vi "Hardware Configuration Dialog.vi"(6 "Update UI Values?":bool, 8 "error in (no error)":errorcluster, 9 "Function":enum16{"Initialize", "Action"}(ring)=enum."Action", 10 "Hardware Status":T1={"Parameter Analyzer"={"Configuration"={"Parameter Analyzer VISA Session"="COM1", "Sweeping Time Parameters"={"Integration Time"=0, "Short Integration Time (s)"=1.0, "Long Integration Time (s)"=0.0, "Wait Time Parameter"=1.0}, "Acquisition Mode"=enum."Sweeping Mode", "Status Polling Time (ms)"=1000, "Comment"="Test VI", "SMU 1 - Sweeping"={"Start / Offset"=0.0, "Stop / Ratio"=1.0, "Step \n(linear only)"=0.01, "Compliance"=0.1, "Power \nCompliance"=0.0, "Mode"=0, "Function"=0, "Sweep Mode"=FALSE}, "SMU 2 - Sweeping"={"Start / Offset"=0.0, "Stop / Ratio"=1.0, "Step \n(linear only)"=0.01, "Compliance"=0.1, "Power \nCompliance"=0.0, "Mode"=0, "Function"=0, "Sweep Mode"=FALSE}, "SMU 3 - Sweeping"={"Start / Offset"=0.0, "Stop / Ratio"=1.0, "Step \n(linear only)"=0.01, "Compliance"=0.1, "Power \nCompliance"=0.0, "Mode"=0, "Function"=0, "Sweep Mode"=FALSE}, "SMU 4 - Sweeping"={"Start / Offset"=0.0, "Stop / Ratio"=1.0, "Step \n(linear only)"=0.01, "Compliance"=0.1, "Power \nCompliance"=0.0, "Mode"=0, "Function"=0, "Sweep Mode"=FALSE}, "Sweep Spacing"=0, "Range"=0, "SMU1 - Sampling"={"Source"=10.0, "Compliance"=1e-05, "Mode"=0, "Function"=FALSE}, "SMU2 - Sampling"={"Source"=10.0, "Compliance"=1e-05, "Mode"=0, "Function"=FALSE}, "SMU3 - Sampling"={"Source"=10.0, "Compliance"=1e-05, "Mode"=0, "Function"=FALSE}, "SMU4 - Sampling"={"Source"=0.1, "Compliance"=60.0, "Mode"=10, "Function"=FALSE}, "Sampling Time Parameters"={"Initial Interval (s)"=0.1, "Number of Samples"=60, "Total Sampling Time (s)"=10.0, "Hold Time (s)"=0.0, "Sampling Mode"=0, "Sampling Time"=0}, "Stop Condition"={"Enable Delay (s)"=0.0, "Name"="", "Threshold"=0.0, "num. of events"=1, "Event"=0, "Stop Condition Enable"=FALSE}}, "Refnums"={"Status"=refnum, "Electrical Measurement"=refnum, "Plots"={"Plot List"=refnum, "Voltage Plot"=refnum, "Current Plot"=refnum, "IV Characteristic"=refnum, "dI/dV-V Characteristic"=refnum}, "HP Integration Time"=refnum, "VISA"=refnum, "Sweeping Time Parameters"=refnum, "Acquisition Mode"=refnum, "SMU 1 - Sweeping"=refnum, "SMU 2 - Sweeping"=refnum, "SMU 3 - Sweeping"=refnum, "SMU 4 - Sweeping"=refnum, "Sweep Spacing"=refnum, "Range"=refnum, "SMU1 - Sampling"=refnum, "SMU2 - Sampling"=refnum, "SMU3 - Sampling"=refnum, "SMU4 - Sampling"=refnum, "Sampling Time Parameters"=refnum, "Stop Condition"=refnum, "Instrument Status"=refnum}, "Initialization"={"Update Visa Session"=FALSE, "Configure Integration Time"=FALSE, "Configure Acquisition Mode"=FALSE, "Update Refnums"=FALSE}}, "Swithing Matrix"={"Configuration"={"Switching Matrix VISA Session"="GPIB0::18::INSTR", "Connections"=[{"Connections"=[FALSE, FALSE, FALSE, FALSE, FALSE, FALSE, FALSE, FALSE, FALSE, FALSE, FALSE, FALSE], "Connection Type"=enum."Disconnected"}, {"Connections"=[FALSE, FALSE, FALSE, FALSE, FALSE, FALSE, FALSE, FALSE, FALSE, FALSE, FALSE, FALSE], "Connection Type"=enum."Disconnected"}, {"Connections"=[FALSE, FALSE, FALSE, FALSE, FALSE, FALSE, FALSE, FALSE, FALSE, FALSE, FALSE, FALSE], "Connection Type"=enum."Disconnected"}, {"Connections"=[FALSE, FALSE, FALSE, FALSE, FALSE, FALSE, FALSE, FALSE, FALSE, FALSE, FALSE, FALSE], "Connection Type"=enum."Disconnected"}, {"Connections"=[FALSE, FALSE, FALSE, FALSE, FALSE, FALSE, FALSE, FALSE, FALSE, FALSE, FALSE, FALSE], "Connection Type"=enum."Disconnected"}, {"Connections"=[FALSE, FALSE, FALSE, FALSE, FALSE, FALSE, FALSE, FALSE, FALSE, FALSE, FALSE, FALSE], "Connection Type"=enum."Disconnected"}, {"Connections"=[FALSE, FALSE, FALSE, FALSE, FALSE, FALSE, FALSE, FALSE, FALSE, FALSE, FALSE, FALSE], "Connection Type"=enum."Disconnected"}, {"Connections"=[FALSE, FALSE, FALSE, FALSE, FALSE, FALSE, FALSE, FALSE, FALSE, FALSE, FALSE, FALSE], "Connection Type"=enum."Disconnected"}]}, "Refnums"={"Connections"=refnum, "Instrument Status"=refnum}, "Initialization"={"Update Visa Session"=FALSE, "Update Refnums"=FALSE}}, "Stress Control"={"Configuration"={"Stress Control VISA Session"="StrainMotor", "Axis"=0, "Motion"=0, "Destination (°)"=0.0, "Speed (°/s)"=4.0, "Position (°)"=25.0}, "Refnums"={"Instrument Status"=refnum, "Position"=refnum, "Mecahnism Motion"=refnum, "Destination"=refnum, "Apply Stress"=refnum, "Stop"=refnum, "Stress Control VISA"=refnum}, "Initialization"={"Update Visa Session"=FALSE, "Update Configuration"=FALSE, "Update Refnums"=FALSE, "Get Position"=FALSE}}, "Optical Spectrometer"={"Configuration"={"Laser Settings"={"Laser Wavelength"=enum."784 nm", "Neutral Density Filter"=enum."50%"}, "Spectrometer Settings"={"Confocal Hole Size (µm)"=150.0, "Grating"=2, "Detector"=enum."InGaAs Array"}, "Acquisition Settings"={"Acquisition Mode"=enum."Multi-Window", "Spectal Position (nm)"=632.0, "From (nm)"=735.0, "To (nm)"=3.0, "Integration Time (s)"=3.0, "Number of Accumulations"=3, "AutoScanning"=FALSE, "Spike Removal"=FALSE}, "Path"=path "C:/07 - Prizes and Awards/Marie Curie Prize/Reply Editors Final NCOMMS(10).docx"}, "Refnums"={"Instrument Status"=refnum, "Optical Spectrum Plot"={"Plot List"=refnum, "Optical Spectrum vs Energy"=refnum, "Optical Spectrum vs Wavelength"=refnum, "Optical Spectrum vs Raman Shift"=refnum, "Detector Temperature"=refnum}, "Laser"=refnum, "Filter"=refnum, "Laser ON?"=refnum, "Hole"=refnum, "Grating"=refnum, "Detector"=refnum, "Acquisition Mode"=refnum, "Spectal Position"=refnum, "From"=refnum, "To"=refnum, "Integration Time"=refnum, "Accumulations"=refnum, "AutoScanning"=refnum, "Spike Removal"=refnum, "Acquisition Mode Panel"=refnum}, "Initialization"={"Connect"=FALSE, "Update Refnums"=FALSE, "Get Configuration"=FALSE}}, "Switches & Mirrors"={"Configuration"={"Relay VISA Session"="COM1", "Switches"={"Laser"=FALSE, "Video"=FALSE}, "Delays (ms)"={"Laser"=500, "Video"=1500}}, "Refnums"={"Instrument Status"=refnum, "Laser"=refnum, "Video"=refnum, "Relay VISA"=refnum}, "Initialize"={"Update Refnums"=FALSE, "Connect"=FALSE, "Set Configuration"=FALSE}}, "Camera"={"Configuration"={"Settings"={"Pixel clock"=20, "Frame rate"=30.0, "Exposure time"=33.21525, "Master Gain"=0, "Red Gain"=0, "Green Gain"=0, "Blue Gain"=0, "Auto Gain"=FALSE, "White-balance"=FALSE, "Color Correction"=FALSE}}, "Refnums"={"Pixel Clock"=refnum, "Frame Rate"=refnum, "Exposure Time"=refnum, "Master Gain"=refnum, "Red Gain"=refnum, "Green Gain"=refnum, "Blue Gain"=refnum, "Auto Gain"=refnum, "Auto White-balance"=refnum, "Color Correction"=refnum, "Image"=refnum, "Video Button"=refnum, "Instrument Status"=refnum}, "Initialization"={"Connect"=FALSE, "Update Refnums"=FALSE, "Acquiring?"=FALSE}}, "XYZ Stage"={"Configuration"={"Connection Settings"={"Tango VISA"="", "Baudrate"=57600, "Show Protocol?"=FALSE}, "Manual Control"={"North"=FALSE, "South"=FALSE, "West"=FALSE, "East"=FALSE, "Up"=FALSE, "Down"=FALSE, "Stop"=FALSE, "XY Step"=0.0, "Z step"=0.0}, "Coordinate Control"={"Motion Mode"=enum."Absolute", "Destination [mm]"=[]}}, "Refnums"={"Instrument Status"=refnum, "Position"=refnum, "Manual Control"=refnum, "Up"=refnum, "Down"=refnum, "North"=refnum, "South"=refnum, "East"=refnum, "West"=refnum, "Stop"=refnum, "Limits"=refnum}, "Initialization"={"Update Visa Session"=FALSE, "Set To Default"=FALSE, "Get Status"=FALSE, "Update Refnums"=FALSE}}, "AutoFocus"={"Configuration"={"Matching Criteria"={"Minimum Score"=700.0, "Color Score Weight"=700.0, "Minimum Contrast"=50, "Match Mode"=0, "Match Feature Mode"=0, "Subpixel Accuracy"=TRUE, "Color Sensitivity"=1, "Search Strategy"=1}, "Z Scan Parameters"={"Z Range"=1380.0, "Resolution"=5000.0, "Initial Direction"=enum."Up", "Focus Threshold"=0.1, "Ascent Constant"=0.1}, "Displacement"=50.0, "Transformation Matrix"=[]}, "Refnums"={"Instrument Status"=refnum, "Matching Criteria"=refnum, "Z Scan Parameters"=refnum, "Distance"=refnum, "Transformation Matrix"=refnum, "Match and Edge"={"Image"=refnum, "Target"=refnum, "Edge"=refnum, "Target Data"=refnum}, "Matching Curves"=refnum, "Tracking"=refnum, "Focus"=refnum, "Find Focus"=refnum, "Set Target"=refnum, "Link Stage & Camera"=refnum, "Align"=refnum}, "Initialize"={"Update Refnums"=FALSE, "Allocate Image Memory"=FALSE, "Set Match Criteria"=FALSE, "Link Stage & Camera"=FALSE, "Set Target"=FALSE, "Find Target"=FALSE}}} {"AutoFocus"."Configuration"."Displacement" scale=1.0..1000.0; "AutoFocus"."Configuration"."Z Scan Parameters"."Focus Threshold" min=0.0 max=1000.0 step=1.0 format="%#_2f"; "AutoFocus"."Configuration"."Z Scan Parameters"."Ascent Constant" min=0.0 max=1000.0 step=1.0 format="%#_2f"; "AutoFocus"."Configuration"."Z Scan Parameters"."Resolution" min=0.0 max=1.0 step=0.01 format="%_2g"; "AutoFocus"."Configuration"."Z Scan Parameters"."Z Range" format="%_3g"; "AutoFocus"."Configuration"."Matching Criteria"."Match Mode" items=["Shift Invariant", "Rotation Invariant"]; "AutoFocus"."Configuration"."Matching Criteria"."Match Feature Mode" items=["Color and Shape", "Color", "Shape"]; "AutoFocus"."Configuration"."Matching Criteria"."Color Sensitivity" items=["Low Sensitivity", "Medium Sensitivity", "High Sensitivity"]; "AutoFocus"."Configuration"."Matching Criteria"."Search Strategy" items=["Conservative", "Balance", "Aggressive", "Very Aggressive"]; "XYZ Stage"."Configuration"."Manual Control"."Z step" scale=0.1..10.0; "XYZ Stage"."Configuration"."Manual Control"."XY Step" scale=0.1..1000.0; "Camera"."Configuration"."Settings"."Blue Gain" min=0 max=100 scale=0.0..100.0; "Camera"."Configuration"."Settings"."Green Gain" min=0 max=100 scale=0.0..100.0; "Camera"."Configuration"."Settings"."Red Gain" min=0 max=100 scale=0.0..100.0; "Camera"."Configuration"."Settings"."Master Gain" min=0 max=100 scale=0.0..100.0; "Camera"."Configuration"."Settings"."Exposure time" min=0.101625 max=159.246375 step=0.101625 scale=0.101625..159.246375 scale format="%#.3g"; "Camera"."Configuration"."Settings"."Frame rate" min=2.7455631699174137 max=6.2675785993528725 step=0.000101625 scale=2.7455631699174137..6.2675785993528725 scale format="%^#_3g"; "Camera"."Configuration"."Settings"."Pixel clock" min=5 max=43 scale=5.0..43.0; "Optical Spectrometer"."Configuration"."Spectrometer Settings"."Grating" items=["1800 l/mm", "150 l/mm"]; "Stress Control"."Configuration"."Axis" min=1 max=3; "Stress Control"."Configuration"."Position (°)" format="%.6g"; "Stress Control"."Configuration"."Speed (°/s)" min=0.0 max=4.0 format="%.6f"; "Stress Control"."Configuration"."Destination (°)" min=-2000000000.0 max=2000000000.0 format="%.6f"; "Stress Control"."Configuration"."Motion" items=["Absolute", "Relative"]; "Parameter Analyzer"."Configuration"."Stop Condition"."Event" items=["Value > Threshold", "Value < Threshold", "| Value | > | Threshold |", "| Value | < | Threshold |"]; "Parameter Analyzer"."Configuration"."Stop Condition"."Threshold" format="%^.2e"; "Parameter Analyzer"."Configuration"."Stop Condition"."Enable Delay (s)" format="%.1f"; "Parameter Analyzer"."Configuration"."Sampling Time Parameters"."Sampling Time" items=["Auto (linear only)", "No Limit", "Set Limit"]; "Parameter Analyzer"."Configuration"."Sampling Time Parameters"."Sampling Mode" items=["Linear", "Log10", "Log25", "Log50", "Thinned Out"]; "Parameter Analyzer"."Configuration"."Sampling Time Parameters"."Hold Time (s)" format="%.4f"; "Parameter Analyzer"."Configuration"."Sampling Time Parameters"."Total Sampling Time (s)" format="%.1f"; "Parameter Analyzer"."Configuration"."Sampling Time Parameters"."Initial Interval (s)" format="%^.3e"; "Parameter Analyzer"."Configuration"."SMU 4 - Sweeping"."Function" items=["Disabled", "Var 1", "Var 2", "Var 1'", "Constant"]; "Parameter Analyzer"."Configuration"."SMU 4 - Sweeping"."Mode" items=["V", "I", "V pulse", "I  pulse", "Common"]; "Parameter Analyzer"."Configuration"."SMU 4 - Sweeping"."Power \nCompliance" format="%^.2e"; "Parameter Analyzer"."Configuration"."SMU 4 - Sweeping"."Compliance" format="%^.2e"; "Parameter Analyzer"."Configuration"."SMU 4 - Sweeping"."Step \n(linear only)" format="%^.4e"; "Parameter Analyzer"."Configuration"."SMU 4 - Sweeping"."Stop / Ratio" format="%^.4e"; "Parameter Analyzer"."Configuration"."SMU 4 - Sweeping"."Start / Offset" format="%^.4e"; "Parameter Analyzer"."Configuration"."SMU 3 - Sweeping"."Function" items=["Disabled", "Var 1", "Var 2", "Var 1'", "Constant"]; "Parameter Analyzer"."Configuration"."SMU 3 - Sweeping"."Mode" items=["V", "I", "V pulse", "I  pulse", "Common"]; "Parameter Analyzer"."Configuration"."SMU 3 - Sweeping"."Power \nCompliance" format="%^.2e"; "Parameter Analyzer"."Configuration"."SMU 3 - Sweeping"."Compliance" format="%^.2e"; "Parameter Analyzer"."Configuration"."SMU 3 - Sweeping"."Step \n(linear only)" format="%^.4e"; "Parameter Analyzer"."Configuration"."SMU 3 - Sweeping"."Stop / Ratio" format="%^.4e"; "Parameter Analyzer"."Configuration"."SMU 3 - Sweeping"."Start / Offset" format="%^.4e"; "Parameter Analyzer"."Configuration"."SMU 2 - Sweeping"."Function" items=["Disabled", "Var 1", "Var 2", "Var 1'", "Constant"]; "Parameter Analyzer"."Configuration"."SMU 2 - Sweeping"."Mode" items=["V", "I", "V pulse", "I  pulse", "Common"]; "Parameter Analyzer"."Configuration"."SMU 2 - Sweeping"."Power \nCompliance" format="%^.2e"; "Parameter Analyzer"."Configuration"."SMU 2 - Sweeping"."Compliance" format="%^.2e"; "Parameter Analyzer"."Configuration"."SMU 2 - Sweeping"."Step \n(linear only)" format="%^.4e"; "Parameter Analyzer"."Configuration"."SMU 2 - Sweeping"."Stop / Ratio" format="%^.4e"; "Parameter Analyzer"."Configuration"."SMU 2 - Sweeping"."Start / Offset" format="%^.4e"; "Parameter Analyzer"."Configuration"."SMU 1 - Sweeping"."Function" items=["Disabled", "Var 1", "Var 2", "Var 1'", "Constant"]; "Parameter Analyzer"."Configuration"."SMU 1 - Sweeping"."Mode" items=["V", "I", "V pulse", "I  pulse", "Common"]; "Parameter Analyzer"."Configuration"."SMU 1 - Sweeping"."Power \nCompliance" format="%^.2e"; "Parameter Analyzer"."Configuration"."SMU 1 - Sweeping"."Compliance" format="%^.2e"; "Parameter Analyzer"."Configuration"."SMU 1 - Sweeping"."Step \n(linear only)" format="%^.4e"; "Parameter Analyzer"."Configuration"."SMU 1 - Sweeping"."Stop / Ratio" format="%^.4e"; "Parameter Analyzer"."Configuration"."SMU 1 - Sweeping"."Start / Offset" format="%^.4e"; "Parameter Analyzer"."Configuration"."Sweeping Time Parameters"."Long Integration Time (s)" scale=0.02..2.0; "Parameter Analyzer"."Configuration"."Sweeping Time Parameters"."Short Integration Time (s)" scale=8e-05..0.00192; "Parameter Analyzer"."Configuration"."Sweeping Time Parameters"."Integration Time" items=["Short", "Long"]; "Parameter Analyzer"."Configuration"."Sweeping Time Parameters"."Wait Time Parameter" format="%.1f"; "Parameter Analyzer"."Configuration"."SMU4 - Sampling"."Mode" items=["V", "I", "Common"]; "Parameter Analyzer"."Configuration"."SMU4 - Sampling"."Compliance" format="%^.2e"; "Parameter Analyzer"."Configuration"."SMU4 - Sampling"."Source" format="%^.3e"; "Parameter Analyzer"."Configuration"."SMU3 - Sampling"."Mode" items=["V", "I", "Common"]; "Parameter Analyzer"."Configuration"."SMU3 - Sampling"."Compliance" format="%^.2e"; "Parameter Analyzer"."Configuration"."SMU3 - Sampling"."Source" format="%^.3e"; "Parameter Analyzer"."Configuration"."SMU2 - Sampling"."Mode" items=["V", "I", "Common"]; "Parameter Analyzer"."Configuration"."SMU2 - Sampling"."Compliance" format="%^.2e"; "Parameter Analyzer"."Configuration"."SMU2 - Sampling"."Source" format="%^.3e"; "Parameter Analyzer"."Configuration"."SMU1 - Sampling"."Mode" items=["V", "I", "Common"]; "Parameter Analyzer"."Configuration"."SMU1 - Sampling"."Compliance" format="%^.2e"; "Parameter Analyzer"."Configuration"."SMU1 - Sampling"."Source" format="%^.3e"; "Parameter Analyzer"."Configuration"."Range" items=["auto", "fixed", "limited"]; "Parameter Analyzer"."Configuration"."Sweep Spacing" items=["linear", "log 10", "log 25", "log 50"]}, 11 "Instrument Steps In":T58) -> (0 "error out":errorcluster, 2 "Instrument Steps Out":T58)   [LabVIEW 2014]
uses:
  Instrument Steps.ctl
  Action.ctl
  Instrument List.ctl
  support/Status of All Instruments.ctl
  Hardware Control/Parameter Analyzer/Parameter Analyzer Data.ctl
  Hardware Control/Parameter Analyzer/Parameter Analyzer Config.ctl
  Hardware Control/Parameter Analyzer/Parameter Analyzer Integration Parameters.ctl
  Hardware Control/Parameter Analyzer/Parameter Analyzer SMU Sweeping.ctl
  Hardware Control/Parameter Analyzer/Parameter Analyzer Sweep Spacing.ctl
  Hardware Control/Parameter Analyzer/Parameter Analyzer SMU Range.ctl
  Hardware Control/Parameter Analyzer/Parameter Analyzer SMU Sampling.ctl
  Hardware Control/Parameter Analyzer/Parameter Analyzer Sampling Parameters.ctl
  Hardware Control/Parameter Analyzer/Parameter Analyzer Stop Sampling Conditions.ctl
  Hardware Control/Parameter Analyzer/Parameter Analyzer Refnums.ctl
  Plot Data/Electrical Data Plot Refnums.ctl
  Hardware Control/Parameter Analyzer/Parameter Analyzer Initialization.ctl
  Hardware Control/Switching Matrix/Switching Matrix Data.ctl
  Hardware Control/Switching Matrix/Switching Matrix Config.ctl
  Hardware Control/Switching Matrix/Switching Matrix Refnums.ctl
  Hardware Control/Switching Matrix/Switching Matrix Initialization.ctl
  Hardware Control/Stress Control/StressControl Data.ctl
  Hardware Control/Stress Control/StressControl Config.ctl
  Hardware Control/Stress Control/StressControl Refnums.ctl
  Hardware Control/Stress Control/StressControl Initialization.ctl
  Hardware Control/Spectrometer/Spectrometer Data.ctl
  Hardware Control/Spectrometer/Spectrometer Config.ctl
  Hardware Control/Spectrometer/Laser Settings.ctl
  Hardware Control/Spectrometer/Laser.ctl
  Hardware Control/Spectrometer/Filter.ctl
  Hardware Control/Spectrometer/Grating Detector Settings.ctl
  Hardware Control/Spectrometer/Grating.ctl
  Hardware Control/Spectrometer/Detector.ctl
  Hardware Control/Spectrometer/Acquisition Settings.ctl
  Hardware Control/Spectrometer/Spectrometer Refnum.ctl
  Plot Data/Optical Spectrum Plot Refnum.ctl
  Hardware Control/Spectrometer/Spectrometer Initialization.ctl
  Hardware Control/Switches and Mirrors/SwitchesMirrors Data.ctl
  Hardware Control/Switches and Mirrors/SwitchesMirrors Config.ctl
  Hardware Control/Switches and Mirrors/SwitchesMirrors Status.ctl
  Hardware Control/Switches and Mirrors/SwitchesMirrors Refnum.ctl
  support/Instrument Status.ctl
  Hardware Control/Switches and Mirrors/SwitchesMirrors Initialize.ctl
  Hardware Control/Camera/Camera Data.ctl
  Hardware Control/Camera/Camera Config.ctl
  Hardware Control/Camera/Camera Settings.ctl
  Hardware Control/Camera/Camera Refnums.ctl
  Hardware Control/Camera/Camera Initialization.ctl
  Hardware Control/XYZ Stage/XYZ Data.ctl
  Hardware Control/XYZ Stage/XYZ Config.ctl
  Hardware Control/XYZ Stage/XYZ Connection Settings.ctl
  Hardware Control/XYZ Stage/XYZ Stage Control.ctl
  Hardware Control/XYZ Stage/XYZ Coordinate Control.ctl
  Hardware Control/XYZ Stage/XYZ Refnums.ctl
  <instrlib>/Tango Drivers/Labview/SubVIs/Axis_Switch.ctl
  Hardware Control/XYZ Stage/XYZ Initialization.ctl
  Hardware Control/Autofocus/AutoFocus Data.ctl
  Hardware Control/Autofocus/AutoFocus Config.ctl
  Hardware Control/Autofocus/ZScan.ctl
  <vilib>/Analysis/Matrix/Datatypes/RealMatrix.ctl
  Hardware Control/Autofocus/AutoFocus Refnums.ctl
  Hardware Control/Autofocus/Target Refnums.ctl
  Hardware Control/Autofocus/AutoFocus Initialize.ctl
  <vilib>/Analysis/Matrix/NI_Matrix.lvlib
panel:
  in  "Unused Functions":enum32{"Delete Step"}(tab)
  in  "Step Index":i32 min=0 max=6 step=1
  in  "Delete Instrument Step":bool
  in  "Action":T61(tab)
  in  "Measure Optoelectronic":bool
  in  "Focus":bool
  in  "Wavelength":T25=enum."365 nm"
  in  "Power":T62(ring)
  in  "Detector":T29=enum."Silicon CCD"
  in  "Grating":T28 items=["1800 l/mm", "150 l/mm"]
  in  "Confocal Hole Size (µm)":dbl=70.0
  in  "Acquisition Mode":enum32{"Single Window", "Multi Window"}(tab)
  in  "Spectal Position (nm)":dbl=363.99945438000003
  in  "From (nm)":dbl=632.0
  in  "To (nm)":dbl=1000.0
  in  "Spectrum Integration Time (s)":dbl=3.0 caption="Integration Time (s)"
  in  "Number of Accumulations":i32=3
  in  "AutoScanning":bool
  in  "Spike Removal":bool
  in  "Configure Spectrometer":bool
  in  "Measure Optical Spectrum":bool
  in  "Switching Matrix Connections":T63(array[cluster])=[{"Connections"=[FALSE, FALSE, FALSE, FALSE, FALSE, FALSE, FALSE, FALSE, FALSE, FALSE, FALSE, FALSE], "Connection Type"=enum."Disconnected"}, {"Connections"=[FALSE, FALSE, FALSE, FALSE, FALSE, FALSE, FALSE, FALSE, FALSE, FALSE, FALSE, FALSE], "Connection Type"=enum."Disconnected"}, {"Connections"=[FALSE, FALSE, FALSE, FALSE, FALSE, FALSE, FALSE, FALSE, FALSE, FALSE, FALSE, FALSE], "Connection Type"=enum."Disconnected"}, {"Connections"=[FALSE, FALSE, FALSE, FALSE, FALSE, FALSE, FALSE, FALSE, FALSE, FALSE, FALSE, FALSE], "Connection Type"=enum."Disconnected"}, {"Connections"=[FALSE, FALSE, FALSE, FALSE, FALSE, FALSE, FALSE, FALSE, FALSE, FALSE, FALSE, FALSE], "Connection Type"=enum."Disconnected"}, {"Connections"=[FALSE, FALSE, FALSE, FALSE, FALSE, FALSE, FALSE, FALSE, FALSE, FALSE, FALSE, FALSE], "Connection Type"=enum."Disconnected"}, {"Connections"=[FALSE, FALSE, FALSE, FALSE, FALSE, FALSE, FALSE, FALSE, FALSE, FALSE, FALSE, FALSE], "Connection Type"=enum."Disconnected"}, {"Connections"=[FALSE, FALSE, FALSE, FALSE, FALSE, FALSE, FALSE, FALSE, FALSE, FALSE, FALSE, FALSE], "Connection Type"=enum."Disconnected"}]
  in  "Configure Switching Matrix":bool
  in  "Measurement Mode":enum32{"Sweeping Mode", "Sampling Mode"}(tab)
  in  "SMU 4 - Sweeping 2":T64={"Start / Offset"=0.0, "Stop / Ratio"=1.0, "Step \n(linear only)"=0.01, "Compliance"=0.1, "Power \nCompliance"=0.0, "Mode"=4, "Function"=4, "Sweep Mode"=FALSE} caption="SMU 4" {"Function" items=["Disabled", "Var 1", "Var 2", "Var 1'", "Constant"]; "Mode" items=["V", "I", "V pulse", "I  pulse", "Common"]; "Power \nCompliance" format="%^.2e"; "Compliance" format="%^.2e"; "Step \n(linear only)" format="%^.4e"; "Stop / Ratio" format="%^.4e"; "Start / Offset" format="%^.4e"}
  in  "SMU 3 - Sweeping 2":T64={"Start / Offset"=0.0, "Stop / Ratio"=1.0, "Step \n(linear only)"=0.01, "Compliance"=0.1, "Power \nCompliance"=0.0, "Mode"=1, "Function"=4, "Sweep Mode"=FALSE} caption="SMU 3" {"Function" items=["Disabled", "Var 1", "Var 2", "Var 1'", "Constant"]; "Mode" items=["V", "I", "V pulse", "I  pulse", "Common"]; "Power \nCompliance" format="%^.2e"; "Compliance" format="%^.2e"; "Step \n(linear only)" format="%^.4e"; "Stop / Ratio" format="%^.4e"; "Start / Offset" format="%^.4e"}
  in  "SMU 2 - Sweeping 2":T64={"Start / Offset"=0.0, "Stop / Ratio"=1.0, "Step \n(linear only)"=0.01, "Compliance"=0.1, "Power \nCompliance"=0.0, "Mode"=1, "Function"=4, "Sweep Mode"=FALSE} caption="SMU 2" {"Function" items=["Disabled", "Var 1", "Var 2", "Var 1'", "Constant"]; "Mode" items=["V", "I", "V pulse", "I  pulse", "Common"]; "Power \nCompliance" format="%^.2e"; "Compliance" format="%^.2e"; "Step \n(linear only)" format="%^.4e"; "Stop / Ratio" format="%^.4e"; "Start / Offset" format="%^.4e"}
  in  "SMU 1 - Sweeping 2":T64={"Start / Offset"=0.0, "Stop / Ratio"=0.15, "Step \n(linear only)"=0.01, "Compliance"=0.1, "Power \nCompliance"=0.0, "Mode"=0, "Function"=1, "Sweep Mode"=TRUE} caption="SMU 1" {"Function" items=["Disabled", "Var 1", "Var 2", "Var 1'", "Constant"]; "Mode" items=["V", "I", "V pulse", "I  pulse", "Common"]; "Power \nCompliance" format="%^.2e"; "Compliance" format="%^.2e"; "Step \n(linear only)" format="%^.4e"; "Stop / Ratio" format="%^.4e"; "Start / Offset" format="%^.4e"}
  in  "User Integration Time":T65={"Integration Time"=0, "Short Integration Time (s)"=0.0, "Long Integration Time (s)"=0.0, "Wait Time Parameter"=1.0} caption="Input Integration Time" {"Long Integration Time (s)" scale=0.02..2.0; "Short Integration Time (s)" scale=8e-05..0.00192; "Integration Time" items=["Short", "Long"]; "Wait Time Parameter" format="%.1f"}
  in  "Range":u16(ring) items=["auto", "fixed", "limited"]
  in  "Sweep Spacing":u16(ring) items=["linear", "log 10", "log 25", "log 50"]
  in  "SMU4 - Sampling":T66={"Source"=10.0, "Compliance"=1e-05, "Mode"=0, "Function"=FALSE} caption="SMU 4" {"Mode" items=["V", "I", "Common"]; "Compliance" format="%^.2e"; "Source" format="%^.3e"}
  in  "SMU2 - Sampling":T66={"Source"=10.0, "Compliance"=1e-05, "Mode"=0, "Function"=FALSE} caption="SMU 2" {"Mode" items=["V", "I", "Common"]; "Compliance" format="%^.2e"; "Source" format="%^.3e"}
  in  "SMU3 - Sampling":T66={"Source"=10.0, "Compliance"=1e-05, "Mode"=0, "Function"=FALSE} caption="SMU 3" {"Mode" items=["V", "I", "Common"]; "Compliance" format="%^.2e"; "Source" format="%^.3e"}
  in  "SMU1 - Sampling":T66={"Source"=10.0, "Compliance"=1e-05, "Mode"=0, "Function"=FALSE} caption="SMU 1" {"Mode" items=["V", "I", "Common"]; "Compliance" format="%^.2e"; "Source" format="%^.3e"}
  in  "Stop Condition":T67={"Enable Delay (s)"=0.0, "Name"="", "Threshold"=0.0, "num. of events"=1, "Event"=0, "Stop Condition Enable"=FALSE} {"Event" items=["Value > Threshold", "Value < Threshold", "| Value | > | Threshold |", "| Value | < | Threshold |"]; "Threshold" format="%^.2e"; "Enable Delay (s)" format="%.1f"}
  in  "Sampling Parameters":T68={"Initial Interval (s)"=0.1, "Number of Samples"=60, "Total Sampling Time (s)"=10.0, "Hold Time (s)"=0.0, "Sampling Mode"=0, "Sampling Time"=0} {"Sampling Time" items=["Auto (linear only)", "No Limit", "Set Limit"]; "Sampling Mode" items=["Linear", "Log10", "Log25", "Log50", "Thinned Out"]; "Hold Time (s)" format="%.4f"; "Total Sampling Time (s)" format="%.1f"; "Initial Interval (s)" format="%^.3e"}
  in  "Configure Generic Parameter Analyzer":bool
  in  "Measure Parameter Analyzer 1":bool
  in  "Integration Time (s)":dbl(slide)=0.02 min=0.02 max=2.0 scale=8e-05..2.0
  in  "Measurement Type":enum32{"Four Probe", "Two Probe"}(ring)
  in  "Force Mode":enum32{"Voltage", "Current"}(ring)
  in  "Power Compliance":dbl format="%^.2e"
  in  "Compliance":dbl=0.001 format="%^.2e"
  in  "Step Size":dbl=0.001 format="%^.4e"
  in  "Maximum Force":dbl=0.15 format="%^.4e"
  in  "Measure Parameter Analyzer 2":bool
  in  "Configure Two/Four Probe":bool
  in  "Sweep Mode":bool
  # "LICENSED MATERIALS – PROPERTY OF IBM\nCopyright IBM Corp. 2016,\nALL RIGHTS RESERVED"
  # "XY"
  # "Z"
  # "XY"
  # "Z"
  # "Laser Settings"
  # "Spectrometer Settings"
  # "Acquisition Settings"
  # "SMU1"
  # "SMU2"
  # "SMU3"
  # "SMU4"
  # "CH1"
  # "CH2"
  # "CH3"
  # "CH4"
  # "L1"
  # "R1"
  # "L2"
  # "R2"
  # "L3"
  # "R3"
  # "L6"
  # "R6"
  # "L7"
  # "R7"
  # "L8"
  # "R8"
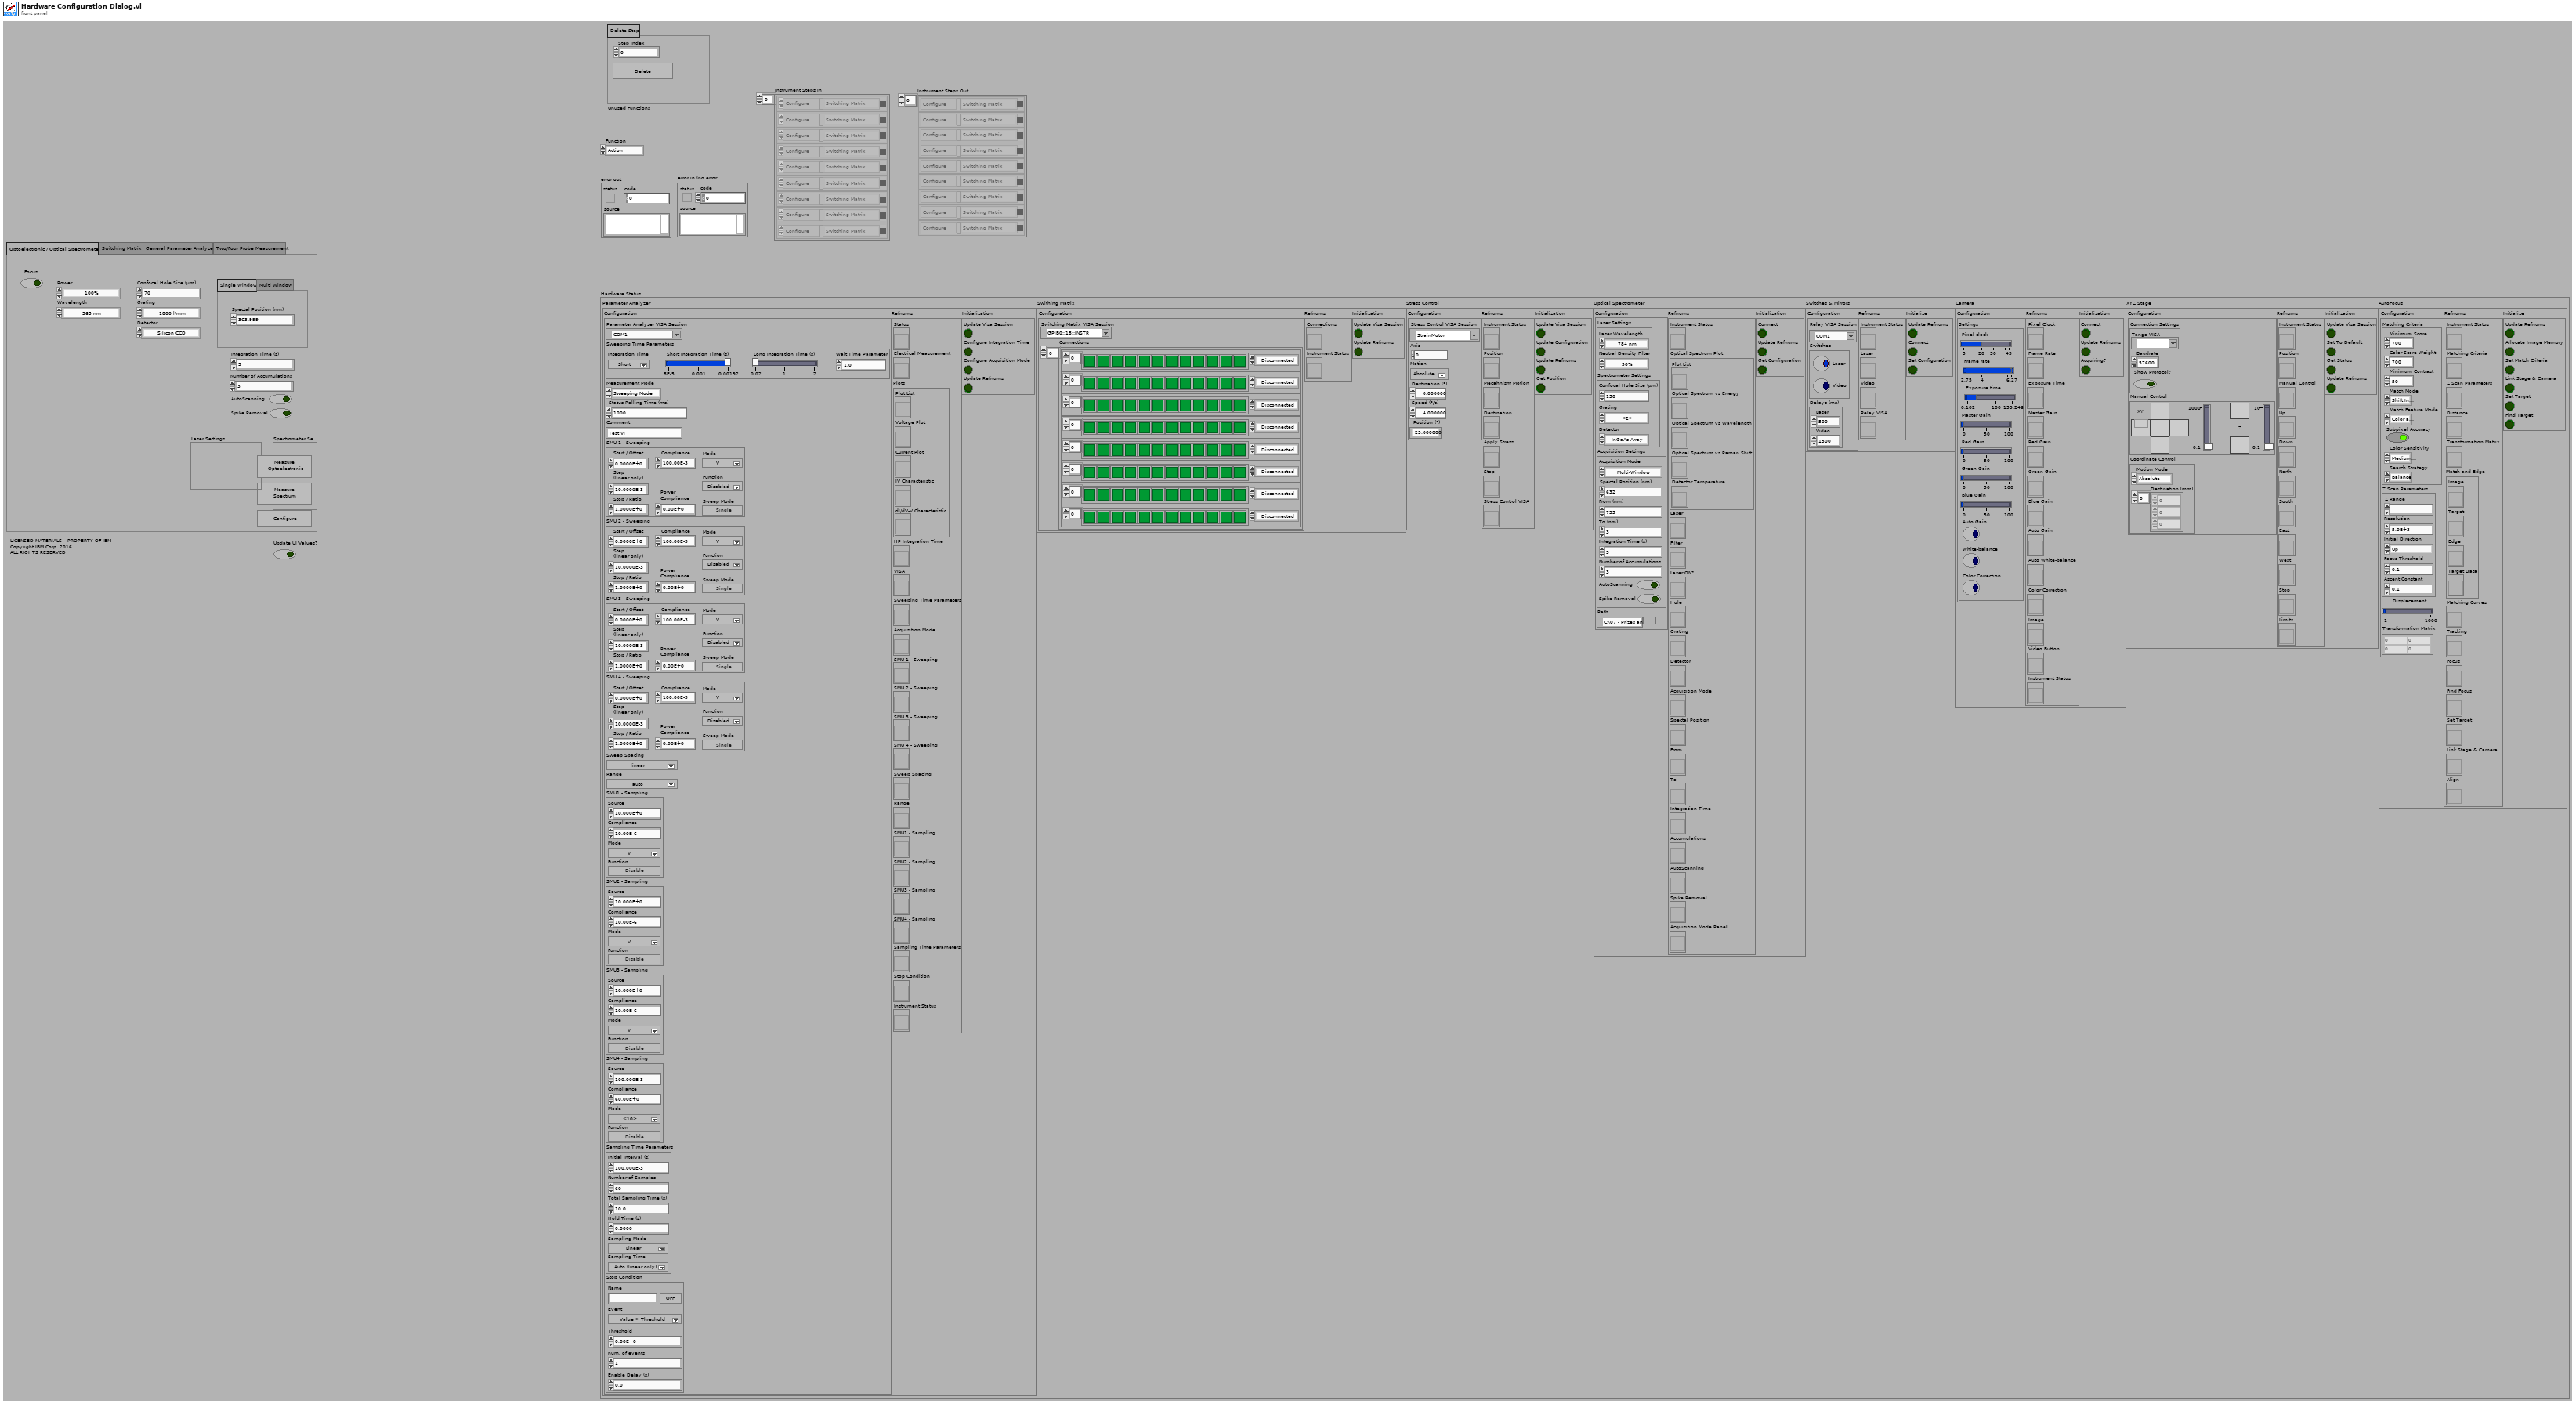
[diagram p1: front panel]
types:
  T1 = typedef "Status of All Instruments.ctl" = cluster{"Parameter Analyzer":T2, "Swithing Matrix":T14, "Stress Control":T18, "Optical Spectrometer":T22, "Switches & Mirrors":T34, "Camera":T39, "XYZ Stage":T44, "AutoFocus":T51}
  T2 = typedef "Parameter Analyzer Data.ctl" = cluster{"Configuration":T3, "Refnums":T11, "Initialization":T13}
  T3 = typedef "Parameter Analyzer Config.ctl" = cluster{"Parameter Analyzer VISA Session":refnum<visa-resource-name>, "Sweeping Time Parameters":T4, "Acquisition Mode":enum32{"Sweeping Mode", "Sampling Mode"}, "Status Polling Time (ms)":u32, "Comment":string, "SMU 1 - Sweeping":T5, "SMU 2 - Sweeping":T5, "SMU 3 - Sweeping":T5, "SMU 4 - Sweeping":T5, "Sweep Spacing":T6, "Range":T7, "SMU1 - Sampling":T8, "SMU2 - Sampling":T8, "SMU3 - Sampling":T8, "SMU4 - Sampling":T8, "Sampling Time Parameters":T9, "Stop Condition":T10}
  T4 = typedef "Parameter Analyzer Integration Parameters.ctl" = cluster{"Integration Time":u32, "Short Integration Time (s)":dbl, "Long Integration Time (s)":dbl, "Wait Time Parameter":dbl}
  T5 = typedef "Parameter Analyzer SMU Sweeping.ctl" = cluster{"Start / Offset":dbl, "Stop / Ratio":dbl, "Step \n(linear only)":dbl, "Compliance":dbl, "Power \nCompliance":dbl, "Mode":u32, "Function":i32, "Sweep Mode":bool}
  T6 = typedef "Parameter Analyzer Sweep Spacing.ctl" = u16
  T7 = typedef "Parameter Analyzer SMU Range.ctl" = u16
  T8 = typedef "Parameter Analyzer SMU Sampling.ctl" = cluster{"Source":dbl, "Compliance":dbl, "Mode":u32, "Function":bool}
  T9 = typedef "Parameter Analyzer Sampling Parameters.ctl" = cluster{"Initial Interval (s)":dbl, "Number of Samples":i32, "Total Sampling Time (s)":dbl, "Hold Time (s)":dbl, "Sampling Mode":i32, "Sampling Time":i32}
  T10 = typedef "Parameter Analyzer Stop Sampling Conditions.ctl" = cluster{"Enable Delay (s)":dbl, "Name":string, "Threshold":dbl, "num. of events":i32, "Event":i32, "Stop Condition Enable":bool}
  T11 = typedef "Parameter Analyzer Refnums.ctl" = cluster{"Status":refnum<vi>, "Electrical Measurement":refnum<vi>, "Plots":T12, "HP Integration Time":refnum<vi>, "VISA":refnum<vi>, "Sweeping Time Parameters":refnum<vi>, "Acquisition Mode":refnum<vi>, "SMU 1 - Sweeping":refnum<vi>, "SMU 2 - Sweeping":refnum<vi>, "SMU 3 - Sweeping":refnum<vi>, "SMU 4 - Sweeping":refnum<vi>, "Sweep Spacing":refnum<vi>, "Range":refnum<vi>, "SMU1 - Sampling":refnum<vi>, "SMU2 - Sampling":refnum<vi>, "SMU3 - Sampling":refnum<vi>, "SMU4 - Sampling":refnum<vi>, "Sampling Time Parameters":refnum<vi>, "Stop Condition":refnum<vi>, "Instrument Status":refnum<vi>}
  T12 = typedef "Electrical Data Plot Refnums.ctl" = cluster{"Plot List":refnum<vi>, "Voltage Plot":refnum<vi>, "Current Plot":refnum<vi>, "IV Characteristic":refnum<vi>, "dI/dV-V Characteristic":refnum<vi>}
  T13 = typedef "Parameter Analyzer Initialization.ctl" = cluster{"Update Visa Session":bool, "Configure Integration Time":bool, "Configure Acquisition Mode":bool, "Update Refnums":bool}
  T14 = typedef "Switching Matrix Data.ctl" = cluster{"Configuration":T15, "Refnums":T16, "Initialization":T17}
  T15 = typedef "Switching Matrix Config.ctl" = cluster{"Switching Matrix VISA Session":refnum<visa-resource-name>, "Connections":cluster{"Connections":bool[], "Connection Type":enum16{"Disconnected", "Make - Break", "Break - Make"}}[]}
  T16 = typedef "Switching Matrix Refnums.ctl" = cluster{"Connections":refnum<vi>, "Instrument Status":refnum<vi>}
  T17 = typedef "Switching Matrix Initialization.ctl" = cluster{"Update Visa Session":bool, "Update Refnums":bool}
  T18 = typedef "StressControl Data.ctl" = cluster{"Configuration":T19, "Refnums":T20, "Initialization":T21}
  T19 = typedef "StressControl Config.ctl" = cluster{"Stress Control VISA Session":refnum<visa-resource-name>, "Axis":i32, "Motion":u16, "Destination (°)":dbl, "Speed (°/s)":dbl, "Position (°)":dbl}
  T20 = typedef "StressControl Refnums.ctl" = cluster{"Instrument Status":refnum<vi>, "Position":refnum<vi>, "Mecahnism Motion":refnum<vi>, "Destination":refnum<vi>, "Apply Stress":refnum<vi>, "Stop":refnum<vi>, "Stress Control VISA":refnum<vi>}
  T21 = typedef "StressControl Initialization.ctl" = cluster{"Update Visa Session":bool, "Update Configuration":bool, "Update Refnums":bool, "Get Position":bool}
  T22 = typedef "Spectrometer Data.ctl" = cluster{"Configuration":T23, "Refnums":T31, "Initialization":T33}
  T23 = typedef "Spectrometer Config.ctl" = cluster{"Laser Settings":T24, "Spectrometer Settings":T27, "Acquisition Settings":T30, "Path":path}
  T24 = typedef "Laser Settings.ctl" = cluster{"Laser Wavelength":T25, "Neutral Density Filter":T26}
  T25 = typedef "Laser.ctl" = enum16{"633 nm", "784 nm", "532 nm", "365 nm"}
  T26 = typedef "Filter.ctl" = enum16{"100%", "50%", "25%", "10%", "1%", "0.1%", "0.01%"}
  T27 = typedef "Grating Detector Settings.ctl" = cluster{"Confocal Hole Size (µm)":dbl, "Grating":T28, "Detector":T29}
  T28 = typedef "Grating.ctl" = u16
  T29 = typedef "Detector.ctl" = enum16{"InGaAs Array", "Silicon CCD"}
  T30 = typedef "Acquisition Settings.ctl" = cluster{"Acquisition Mode":enum16{"Single Window", "Multi-Window"}, "Spectal Position (nm)":dbl, "From (nm)":dbl, "To (nm)":dbl, "Integration Time (s)":dbl, "Number of Accumulations":i32, "AutoScanning":bool, "Spike Removal":bool}
  T31 = typedef "Spectrometer Refnum.ctl" = cluster{"Instrument Status":refnum<vi>, "Optical Spectrum Plot":T32, "Laser":refnum<vi>, "Filter":refnum<vi>, "Laser ON?":refnum<vi>, "Hole":refnum<vi>, "Grating":refnum<vi>, "Detector":refnum<vi>, "Acquisition Mode":refnum<vi>, "Spectal Position":refnum<vi>, "From":refnum<vi>, "To":refnum<vi>, "Integration Time":refnum<vi>, "Accumulations":refnum<vi>, "AutoScanning":refnum<vi>, "Spike Removal":refnum<vi>, "Acquisition Mode Panel":refnum<vi>}
  T32 = typedef "Optical Spectrum Plot Refnum.ctl" = cluster{"Plot List":refnum<vi>, "Optical Spectrum vs Energy":refnum<vi>, "Optical Spectrum vs Wavelength":refnum<vi>, "Optical Spectrum vs Raman Shift":refnum<vi>, "Detector Temperature":refnum<vi>}
  T33 = typedef "Spectrometer Initialization.ctl" = cluster{"Connect":bool, "Update Refnums":bool, "Get Configuration":bool}
  T34 = typedef "SwitchesMirrors Data.ctl" = cluster{"Configuration":T35, "Refnums":T37, "Initialize":T38}
  T35 = typedef "SwitchesMirrors Config.ctl" = cluster{"Relay VISA Session":refnum<visa-resource-name>, "Switches":T36, "Delays (ms)":cluster{"Laser":u32, "Video":u32}}
  T36 = typedef "SwitchesMirrors Status.ctl" = cluster{"Laser":bool, "Video":bool}
  T37 = typedef "SwitchesMirrors Refnum.ctl" = cluster{"Instrument Status":refnum<vi>, "Laser":refnum<vi>, "Video":refnum<vi>, "Relay VISA":refnum<vi>}
  T38 = typedef "SwitchesMirrors Initialize.ctl" = cluster{"Update Refnums":bool, "Connect":bool, "Set Configuration":bool}
  T39 = typedef "Camera Data.ctl" = cluster{"Configuration":T40, "Refnums":T42, "Initialization":T43}
  T40 = typedef "Camera Config.ctl" = cluster{"Settings":T41}
  T41 = typedef "Camera Settings.ctl" = cluster{"Pixel clock":i32, "Frame rate":dbl, "Exposure time":dbl, "Master Gain":i32, "Red Gain":i32, "Green Gain":i32, "Blue Gain":i32, "Auto Gain":bool, "White-balance":bool, "Color Correction":bool}
  T42 = typedef "Camera Refnums.ctl" = cluster{"Pixel Clock":refnum<vi>, "Frame Rate":refnum<vi>, "Exposure Time":refnum<vi>, "Master Gain":refnum<vi>, "Red Gain":refnum<vi>, "Green Gain":refnum<vi>, "Blue Gain":refnum<vi>, "Auto Gain":refnum<vi>, "Auto White-balance":refnum<vi>, "Color Correction":refnum<vi>, "Image":refnum<vi>, "Video Button":refnum<vi>, "Instrument Status":refnum<vi>}
  T43 = typedef "Camera Initialization.ctl" = cluster{"Connect":bool, "Update Refnums":bool, "Acquiring?":bool}
  T44 = typedef "XYZ Data.ctl" = cluster{"Configuration":T45, "Refnums":T49, "Initialization":T50}
  T45 = typedef "XYZ Config.ctl" = cluster{"Connection Settings":T46, "Manual Control":T47, "Coordinate Control":T48}
  T46 = typedef "XYZ Connection Settings.ctl" = cluster{"Tango VISA":refnum<visa-resource-name>, "Baudrate":i32, "Show Protocol?":bool}
  T47 = typedef "XYZ Stage Control.ctl" = cluster{"North":bool, "South":bool, "West":bool, "East":bool, "Up":bool, "Down":bool, "Stop":bool, "XY Step":dbl, "Z step":dbl}
  T48 = typedef "XYZ Coordinate Control.ctl" = cluster{"Motion Mode":enum16{"Absolute", "Relative"}, "Destination [mm]":dbl[]}
  T49 = typedef "XYZ Refnums.ctl" = cluster{"Instrument Status":refnum<vi>, "Position":refnum<vi>, "Manual Control":refnum<vi>, "Up":refnum<vi>, "Down":refnum<vi>, "North":refnum<vi>, "South":refnum<vi>, "East":refnum<vi>, "West":refnum<vi>, "Stop":refnum<vi>, "Limits":refnum<vi>}
  T50 = typedef "XYZ Initialization.ctl" = cluster{"Update Visa Session":bool, "Set To Default":bool, "Get Status":bool, "Update Refnums":bool}
  T51 = typedef "AutoFocus Data.ctl" = cluster{"Configuration":T52, "Refnums":T55, "Initialize":T57}
  T52 = typedef "AutoFocus Config.ctl" = cluster{"Matching Criteria":cluster{"Minimum Score":sgl, "Color Score Weight":sgl, "Minimum Contrast":i32, "Match Mode":u32, "Match Feature Mode":u32, "Subpixel Accuracy":bool, "Color Sensitivity":u32, "Search Strategy":u32}, "Z Scan Parameters":T53, "Displacement":dbl, "Transformation Matrix":T54}
  T53 = typedef "ZScan.ctl" = cluster{"Z Range":ext, "Resolution":dbl, "Initial Direction":enum16{"Up", "Down"}, "Focus Threshold":dbl, "Ascent Constant":dbl}
  T54 = typedef "NI_Matrix.lvlib/RealMatrix.ctl" = dbl[][]
  T55 = typedef "AutoFocus Refnums.ctl" = cluster{"Instrument Status":refnum<vi>, "Matching Criteria":refnum<vi>, "Z Scan Parameters":refnum<vi>, "Distance":refnum<vi>, "Transformation Matrix":refnum<vi>, "Match and Edge":T56, "Matching Curves":refnum<vi>, "Tracking":refnum<vi>, "Focus":refnum<vi>, "Find Focus":refnum<vi>, "Set Target":refnum<vi>, "Link Stage & Camera":refnum<vi>, "Align":refnum<vi>}
  T56 = typedef "Target Refnums.ctl" = cluster{"Image":refnum<vi>, "Target":refnum<vi>, "Edge":refnum<vi>, "Target Data":refnum<vi>}
  T57 = typedef "AutoFocus Initialize.ctl" = cluster{"Update Refnums":bool, "Allocate Image Memory":bool, "Set Match Criteria":bool, "Link Stage & Camera":bool, "Set Target":bool, "Find Target":bool}
  T58 = typedef "Instrument Steps.ctl" = cluster{"Action":T59, "Configuration":variant, "Instrument":T60, "Status":enum8{"False", "True", "Mixed"}}[]
  T59 = typedef "Action.ctl" = enum32{"Configure", "Measure"}
  T60 = typedef "Instrument List.ctl" = enum32{"Unknown Instrument", "Switching Matrix", "Parameter Analyzer", "Optical Spectrometer", "Optoelectronic", "Autofocus"}
  T61 = enum32{"Optoelectronic / Optical Spectrometer", "Switching Matrix", "General Parameter Analyzer", "Two/Four Probe Measurement"}
  T62 = enum16{"100%", "50%", "25%", "10%", "1%", "0.1%", "0.01%", "OFF"}
  T63 = cluster{"Connections":bool[], "Connection Type":enum16{"Disconnected", "Make - Break", "Break - Make"}}[]
  T64 = cluster{"Start / Offset":dbl, "Stop / Ratio":dbl, "Step \n(linear only)":dbl, "Compliance":dbl, "Power \nCompliance":dbl, "Mode":u32, "Function":i32, "Sweep Mode":bool}
  T65 = cluster{"Integration Time":u32, "Short Integration Time (s)":dbl, "Long Integration Time (s)":dbl, "Wait Time Parameter":dbl}
  T66 = cluster{"Source":dbl, "Compliance":dbl, "Mode":u32, "Function":bool}
  T67 = cluster{"Enable Delay (s)":dbl, "Name":string, "Threshold":dbl, "num. of events":i32, "Event":i32, "Stop Condition Enable":bool}
  T68 = cluster{"Initial Interval (s)":dbl, "Number of Samples":i32, "Total Sampling Time (s)":dbl, "Hold Time (s)":dbl, "Sampling Mode":i32, "Sampling Time":i32}
  T69 = enum8{"Enabled", "Disabled", "Disabled and Grayed Out"}
  T70 = cluster{"Measurement Type":enum32{"Four Probe", "Two Probe"}, "Sweep Mode":bool, "Force Mode":enum32{"Voltage", "Current"}, "Maximum Force":dbl, "Step Size":dbl, "Compliance":dbl, "Power Compliance":dbl, "Integration Time (s)":dbl}
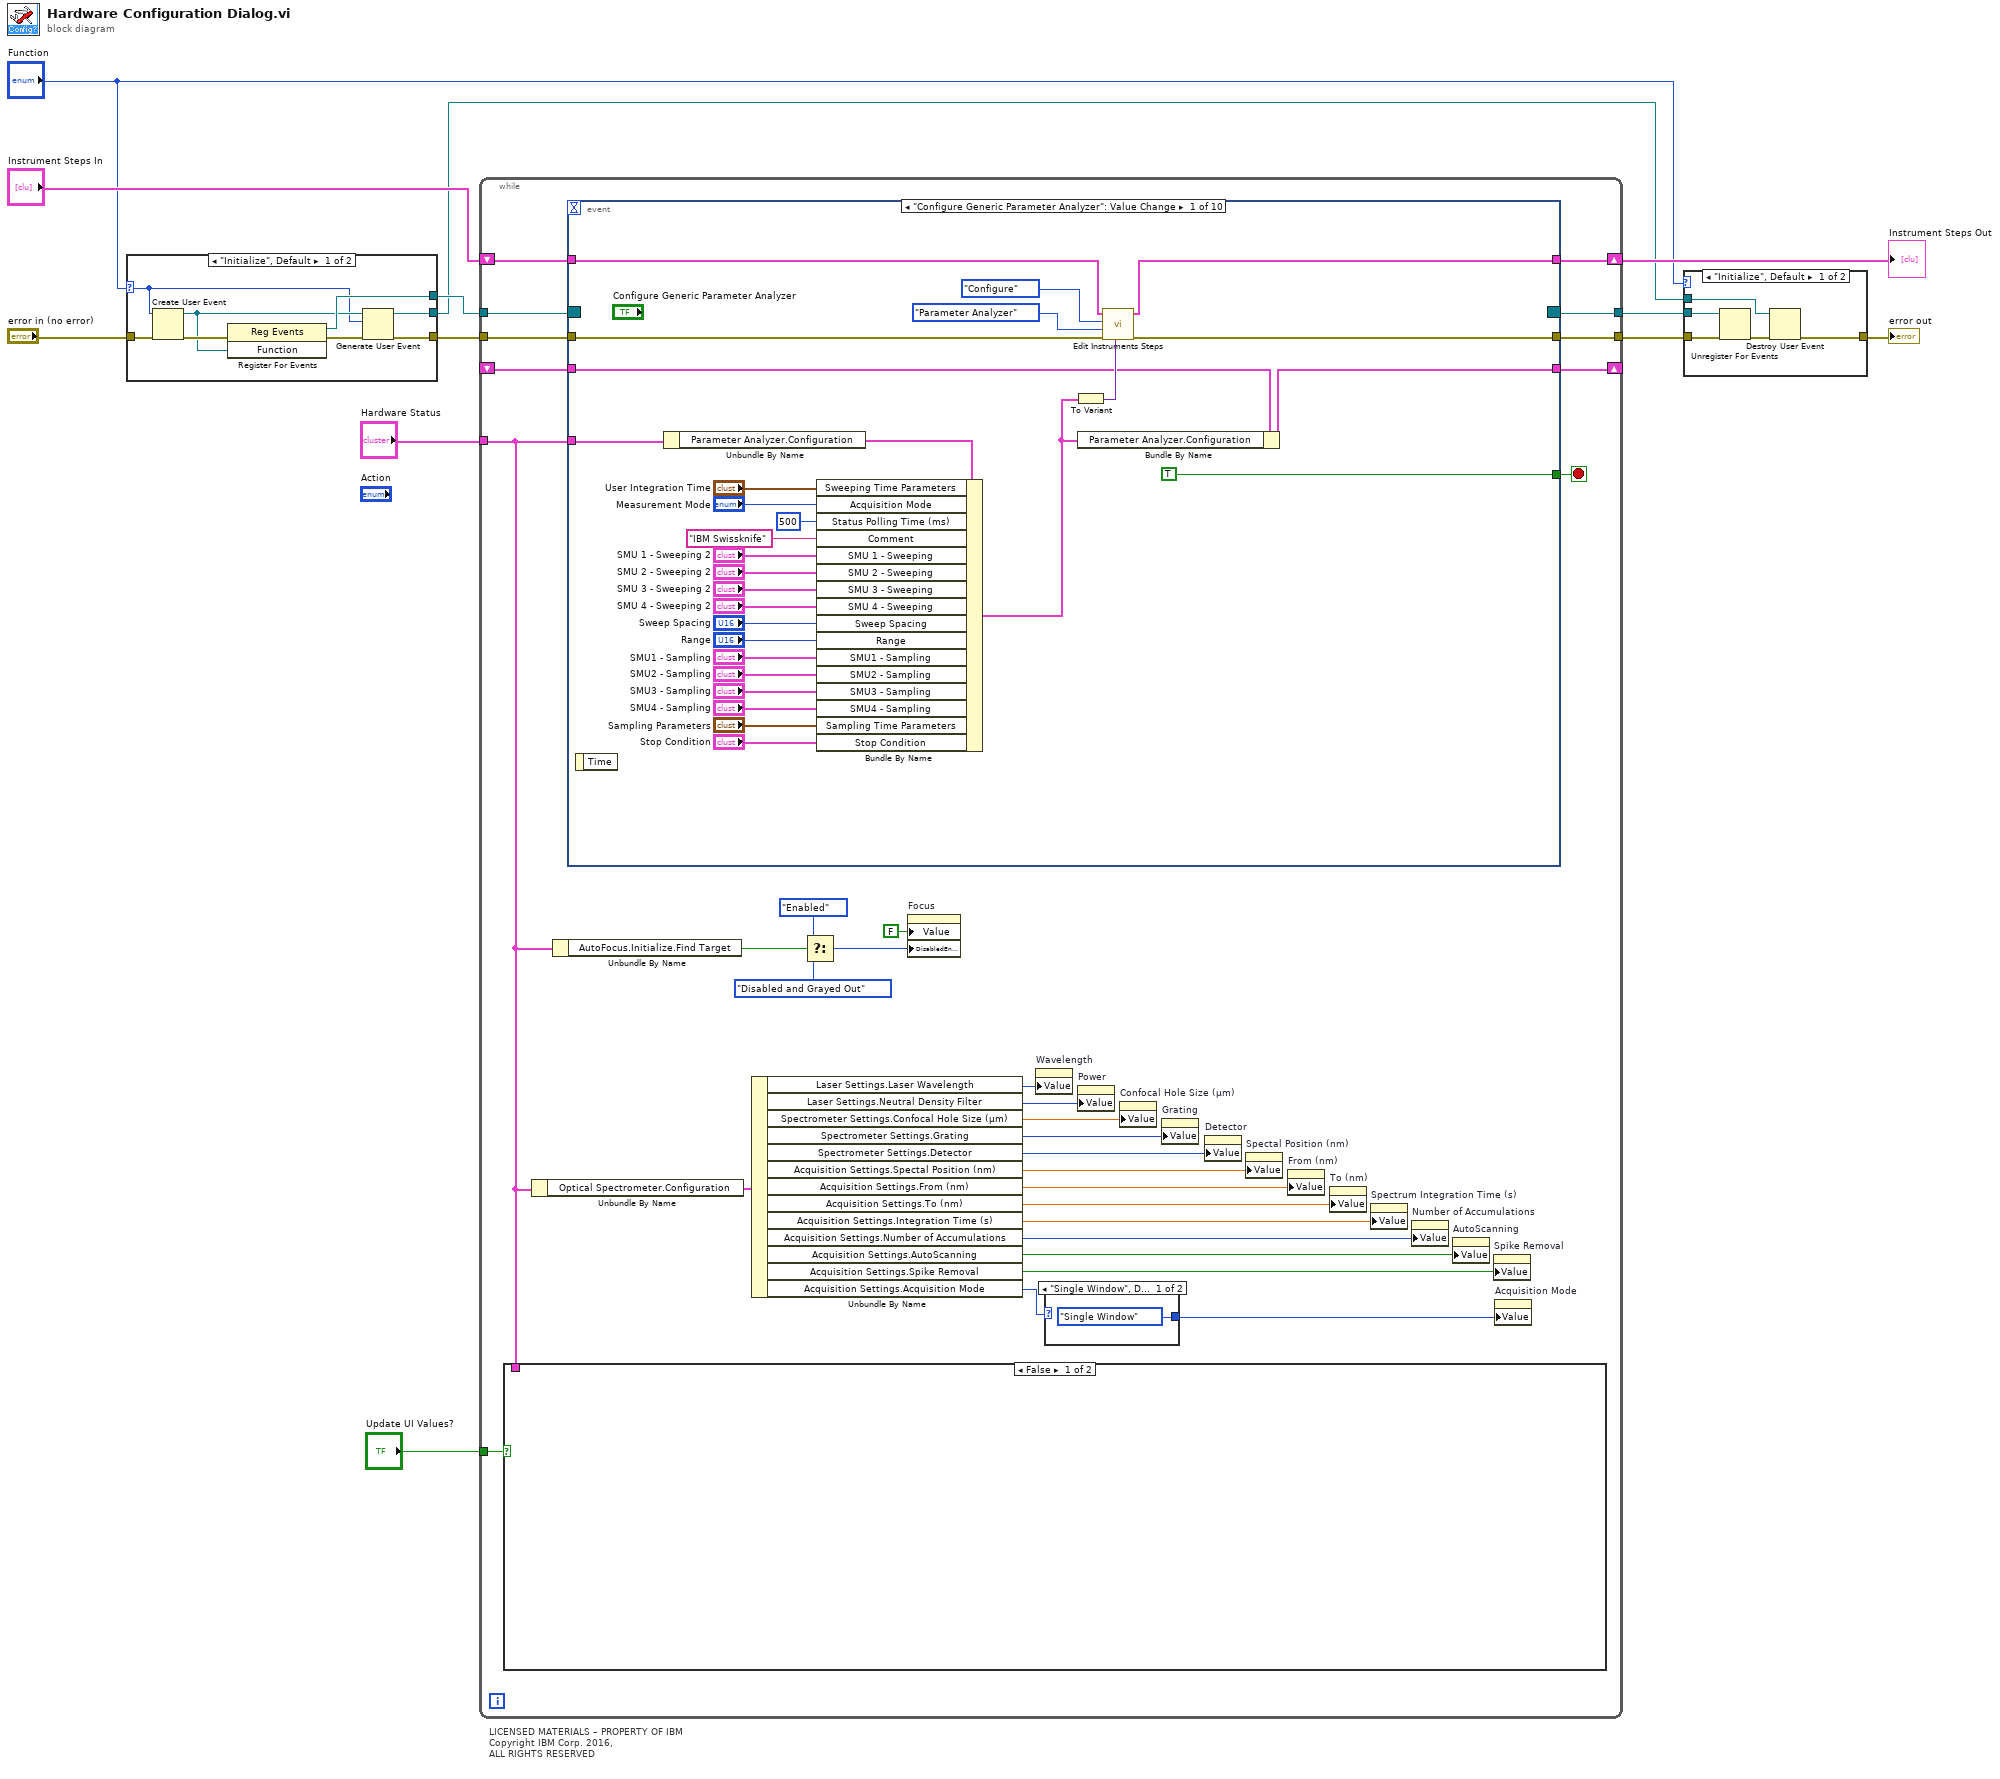
[diagram p0: block diagram]
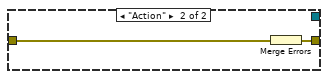
[diagram p3: hidden frame]
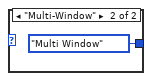
[diagram p4: hidden frame]
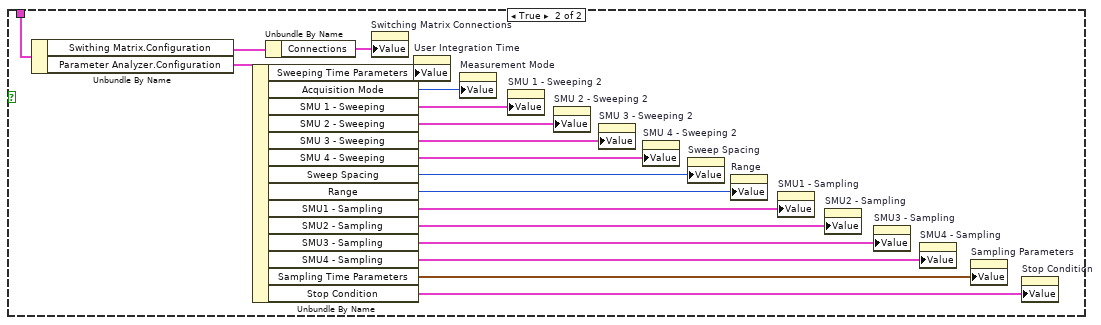
[diagram p5: hidden frame]
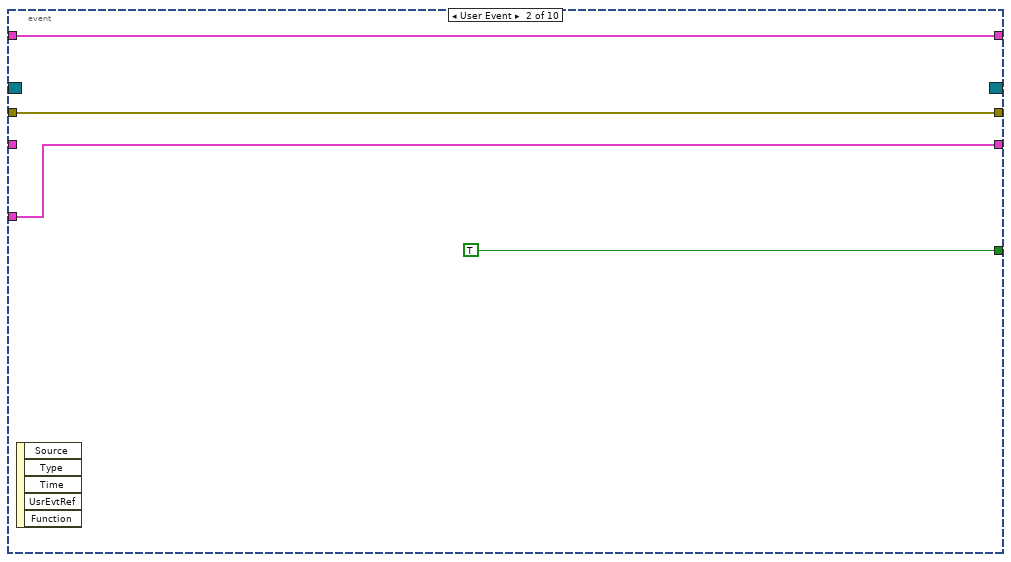
[diagram p6: hidden frame]
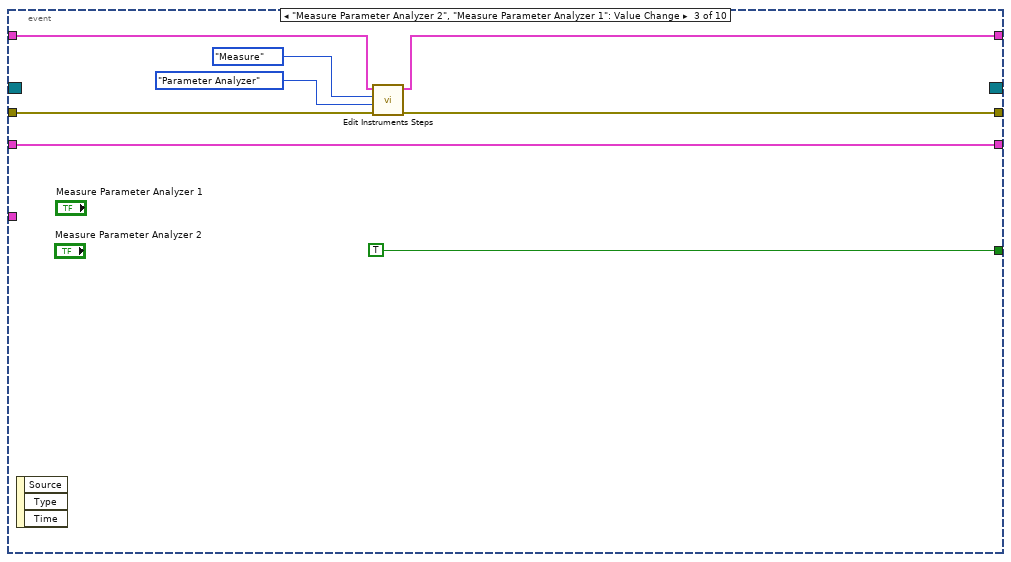
[diagram p7: hidden frame]
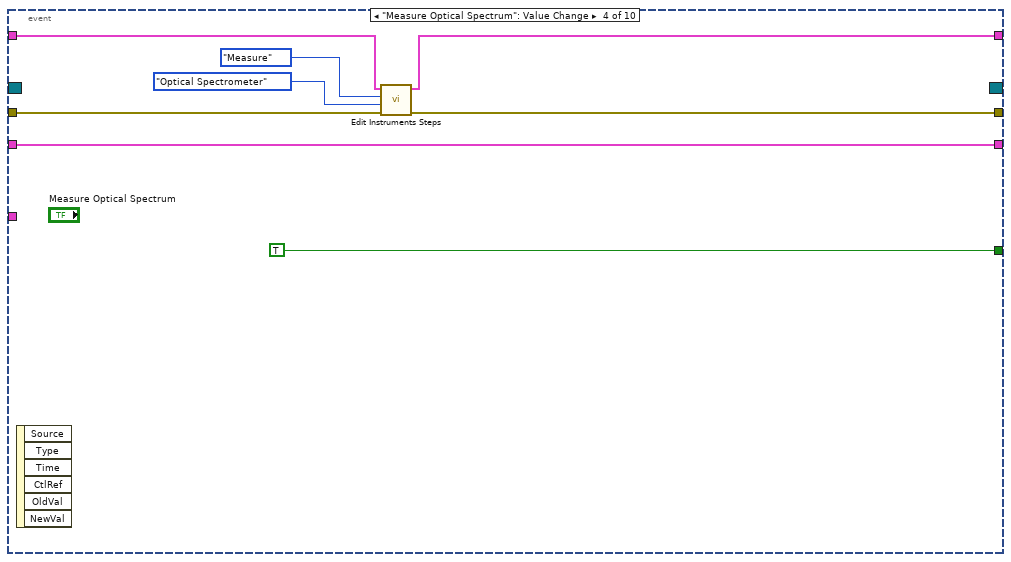
[diagram p8: hidden frame]
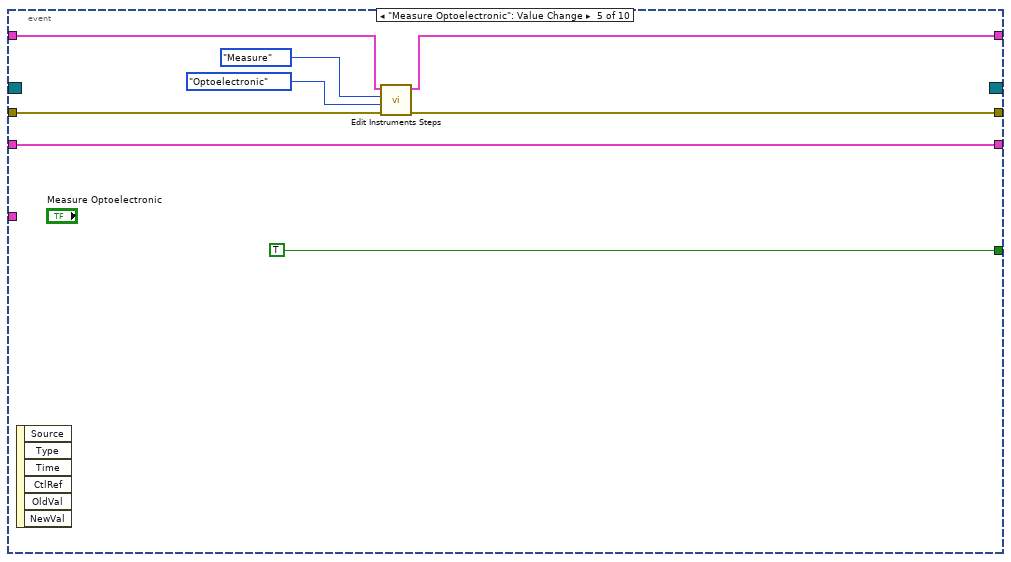
[diagram p9: hidden frame]
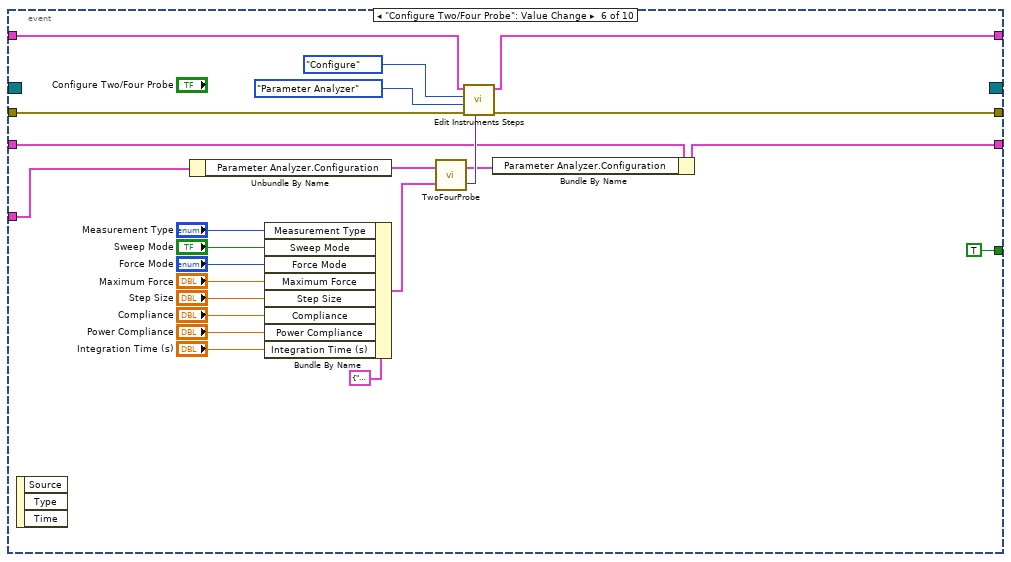
[diagram p10: hidden frame]
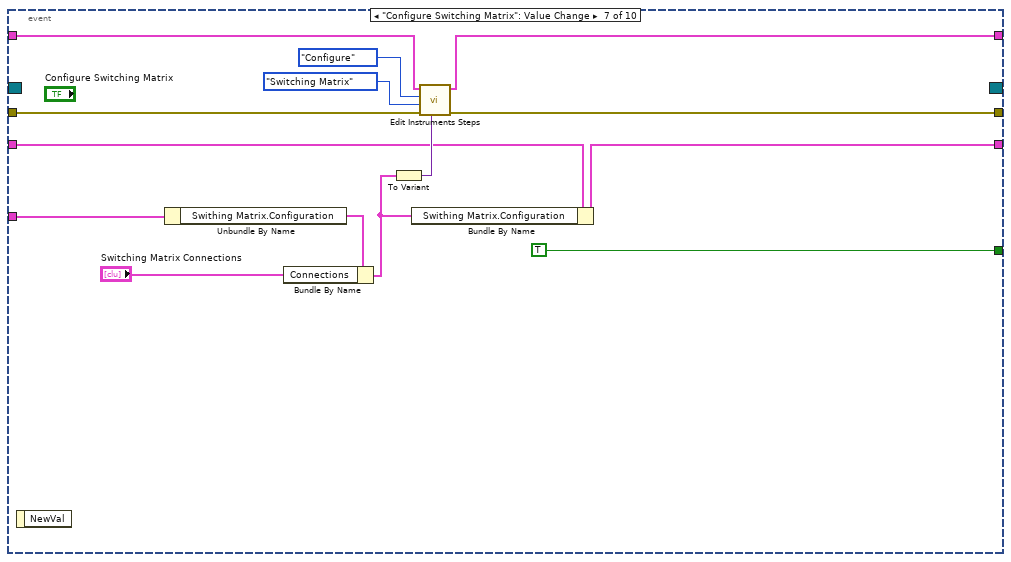
[diagram p11: hidden frame]
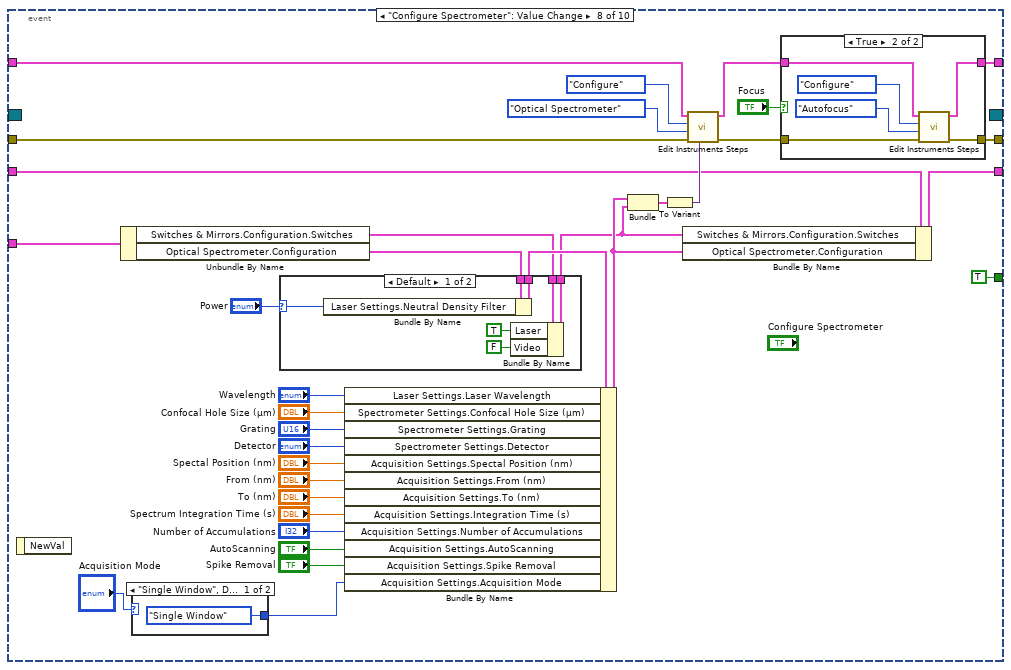
[diagram p12: hidden frame]
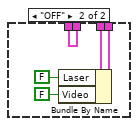
[diagram p14: hidden frame]
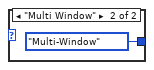
[diagram p15: hidden frame]
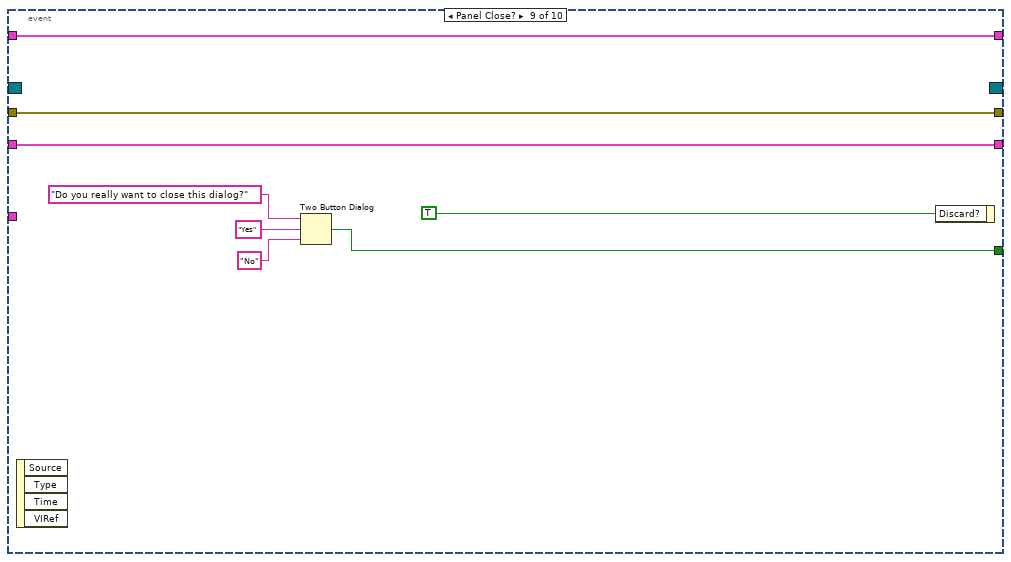
[diagram p16: hidden frame]
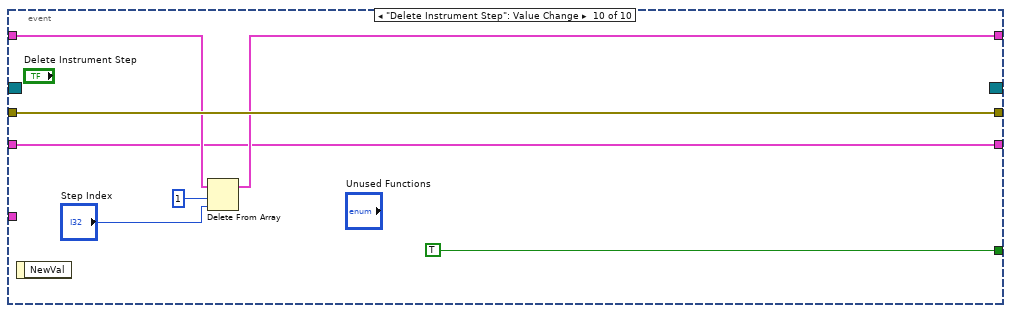
[diagram p17: hidden frame]
diagram:
  # "LICENSED MATERIALS – PROPERTY OF IBM\nCopyright IBM Corp. 2016,\nALL RIGHTS RESERVED"
  n1 = case shown="\"Initialize\", Default" "Function" {
    selector: "Function" -> [w15 _]
    tunnel: [w20 _] -> w9
    tunnel: [w13 w22] -> w8
    tunnel: "error in (no error)" -> [w14 w21]
    tunnel: [w16 _] -> w2
    frame "Initialize", Default {
      n2 = Create User Event(user event datatype=w15, error in=w14) -> (user event=w18:refnum<user-event>, error out=w19:errorcluster)
      n3 = register-events(error in=w19, w18) -> (reference out=w20:refnum<event-registration>, error out=w17:errorcluster)  [unwired: 1 in]
      n4 = Generate User Event(user event=w18, event data cluster=w15, error in=w17) -> (user event out=w16:refnum<user-event>, error out=w13:errorcluster)  [unwired: 1 in]
    }
    frame "Action" {
      n5 = Merge Errors(w21) -> (w22:errorcluster)
    }
  }
  n6 = while {
    tunnel: [w52] -> w6
    tunnel: w8 -> [w51]
    shift-right: [w49] -> w11
    shift-left: "Instrument Steps In" -> [w50]
    shift-right: [w39] -> _
    shift-left: _ -> [w45]
    tunnel: "Hardware Status" -> [w38]
    tunnel: w9 -> [w48]
    tunnel: [w47] -> w3
    tunnel: "Update UI Values?" -> [w46]
    stop <- w53 stop-if-true
    n7 = case shown="False" w46 {
      tunnel: w38 -> [_ w56]
      frame False {
      }
      frame True {
        n8 = Unbundle By Name(w56) -> ("Swithing Matrix.Configuration"=w57:T15, "Parameter Analyzer.Configuration"=w58:T3)
        n9 = Unbundle By Name(w58) -> ("Sweeping Time Parameters"=w73:T4, "Acquisition Mode"=w72:enum32{"Sweeping Mode", "Sampling Mode"}, "SMU 1 - Sweeping"=w69:T5, "SMU 2 - Sweeping"=w68:T5, "SMU 3 - Sweeping"=w67:T5, "SMU 4 - Sweeping"=w66:T5, "Sweep Spacing"=w71:T6, "Range"=w70:T7, "SMU1 - Sampling"=w65:T8, "SMU2 - Sampling"=w64:T8, "SMU3 - Sampling"=w63:T8, "SMU4 - Sampling"=w62:T8, "Sampling Time Parameters"=w61:T9, "Stop Condition"=w60:T10)
        n10 = Unbundle By Name(w57) -> ("Connections"=w59:T63)
        n11 = property on="Switching Matrix Connections" class="Arr (strict)"("Value"=w59) -> ()  [unwired: 2 in, 2 out]
        n12 = property on="User Integration Time" class="Clust (strict)"("Value"=w73) -> ()  [unwired: 2 in, 2 out]
        n13 = property on="Measurement Mode" class="TabCtl (strict)"("Value"=w72) -> ()  [unwired: 2 in, 2 out]
        n14 = property on="SMU 1 - Sweeping 2" class="Clust (strict)"("Value"=w69) -> ()  [unwired: 2 in, 2 out]
        n15 = property on="SMU 2 - Sweeping 2" class="Clust (strict)"("Value"=w68) -> ()  [unwired: 2 in, 2 out]
        n16 = property on="SMU 3 - Sweeping 2" class="Clust (strict)"("Value"=w67) -> ()  [unwired: 2 in, 2 out]
        n17 = property on="SMU 4 - Sweeping 2" class="Clust (strict)"("Value"=w66) -> ()  [unwired: 2 in, 2 out]
        n18 = property on="Sweep Spacing" class="Ring (strict)"("Value"=w71) -> ()  [unwired: 2 in, 2 out]
        n19 = property on="Range" class="Ring (strict)"("Value"=w70) -> ()  [unwired: 2 in, 2 out]
        n20 = property on="SMU1 - Sampling" class="Clust (strict)"("Value"=w65) -> ()  [unwired: 2 in, 2 out]
        n21 = property on="SMU2 - Sampling" class="Clust (strict)"("Value"=w64) -> ()  [unwired: 2 in, 2 out]
        n22 = property on="SMU3 - Sampling" class="Clust (strict)"("Value"=w63) -> ()  [unwired: 2 in, 2 out]
        n23 = property on="SMU4 - Sampling" class="Clust (strict)"("Value"=w62) -> ()  [unwired: 2 in, 2 out]
        n24 = property on="Sampling Parameters" class="Clust (strict)"("Value"=w61) -> ()  [unwired: 2 in, 2 out]
        n25 = property on="Stop Condition" class="Clust (strict)"("Value"=w60) -> ()  [unwired: 2 in, 2 out]
      }
    }
    n26 = Unbundle By Name(w38) -> ("Optical Spectrometer.Configuration"=w23:T23)
    n27 = Unbundle By Name(w38) -> ("AutoFocus.Initialize.Find Target"=w44:bool)
    n28 = event shown="[0] \"Configure Generic Parameter Analyzer\": Value Change" {
      selector: w48 -> [_ _ _ _ _ _ _ _ _ _]
      dyn-events: [_ _ _ _ _ _ _ _ _ _] -> w47
      timeout: _ -> [_ _ _ _ _ _ _ _ _ _]
      tunnel: [TRUE ("T button?") TRUE ("T button?") TRUE ("T button?") TRUE ("T button?") TRUE ("T button?") TRUE ("T button?") TRUE ("T button?") TRUE ("T button?") w228 TRUE ("T button?")] -> w53
      tunnel: [w82 w106 w111 w117 w125 w150 w162 w171 w227 w237] -> w52
      tunnel: w51 -> [w76 w106 w112 w116 w124 w149 w161 w172 w227 w237]
      tunnel: w50 -> [w81 w105 w110 w119 w127 w148 w159 w168 w226 w235]
      tunnel: [w80 w105 w109 w118 w126 w147 w160 w170 w226 w234] -> w49
      tunnel: w38 -> [w77 w104 _ _ _ w145 w157 w196 _ _]
      tunnel: [w75 w104 w107 w120 w128 w143 w155 w194 w225 w232] -> w39
      tunnel: w45 -> [w74 _ w107 w120 w128 w144 w156 w195 w225 w232]
      event "Configure Generic Parameter Analyzer": Value Change {
        n29 = event-data() -> ()  [unwired: 2 out]
        n30 = Unbundle By Name(w77) -> ("Parameter Analyzer.Configuration"=w102:T3)
        n31 = Bundle By Name(cluster=w102, "Sweeping Time Parameters"="User Integration Time", "Acquisition Mode"="Measurement Mode", "Status Polling Time (ms)"=u32 500, "Comment"="IBM Swissknife", "SMU 1 - Sweeping"="SMU 1 - Sweeping 2", "SMU 2 - Sweeping"="SMU 2 - Sweeping 2", "SMU 3 - Sweeping"="SMU 3 - Sweeping 2", "SMU 4 - Sweeping"="SMU 4 - Sweeping 2", "Sweep Spacing"="Sweep Spacing", "Range"="Range", "SMU1 - Sampling"="SMU1 - Sampling", "SMU2 - Sampling"="SMU2 - Sampling", "SMU3 - Sampling"="SMU3 - Sampling", "SMU4 - Sampling"="SMU4 - Sampling", "Sampling Time Parameters"="Sampling Parameters", "Stop Condition"="Stop Condition") -> (w78:T3)
        n32 = To Variant(anything=w78) -> (Variant=w85:variant)
        n33 = Bundle By Name(cluster=w74, "Parameter Analyzer.Configuration"=w78) -> (w75:T1)
        n34 = call "Edit Instruments Steps.vi"("Configuration"=w85, "error in (no error)"=w76, "Instrument"=Instrument_List."Parameter Analyzer", "Action"=Action."Configure", "Instrument Steps In"=w81) -> ("error out"=w82:errorcluster, "Instrument Steps Out"=w80:T58)  [unwired: 2 in, 2 out]
      }
      event User Event {
        n35 = event-data() -> ()  [unwired: 6 out]
      }
      event "Measure Parameter Analyzer 2", "Measure Parameter Analyzer 1": Value Change {
        n36 = event-data() -> ()  [unwired: 4 out]
        n37 = call "Edit Instruments Steps.vi"("error in (no error)"=w112, "Instrument"=Instrument_List."Parameter Analyzer", "Action"=Action."Measure", "Instrument Steps In"=w110) -> ("error out"=w111:errorcluster, "Instrument Steps Out"=w109:T58)  [unwired: 3 in, 2 out]
      }
      event "Measure Optical Spectrum": Value Change {
        n38 = event-data() -> ()  [unwired: 7 out]
        n39 = call "Edit Instruments Steps.vi"("error in (no error)"=w116, "Instrument"=Instrument_List."Optical Spectrometer", "Action"=Action."Measure", "Instrument Steps In"=w119) -> ("error out"=w117:errorcluster, "Instrument Steps Out"=w118:T58)  [unwired: 3 in, 2 out]
      }
      event "Measure Optoelectronic": Value Change {
        n40 = event-data() -> ()  [unwired: 7 out]
        n41 = call "Edit Instruments Steps.vi"("error in (no error)"=w124, "Instrument"=Instrument_List."Optoelectronic", "Action"=Action."Measure", "Instrument Steps In"=w127) -> ("error out"=w125:errorcluster, "Instrument Steps Out"=w126:T58)  [unwired: 3 in, 2 out]
      }
      event "Configure Two/Four Probe": Value Change {
        n42 = event-data() -> ()  [unwired: 4 out]
        n43 = Unbundle By Name(w145) -> ("Parameter Analyzer.Configuration"=w132:T3)
        n44 = Bundle By Name(cluster=T70 {"Measurement Type"=enum."Four Probe", "Sweep Mode"=FALSE, "Force Mode"=enum."Voltage", "Maximum Force"=0.0, "Step Size"=0.0, "Compliance"=0.0, "Power Compliance"=0.0, "Integration Time (s)"=0.0} ("Sweeping Measurement"), "Measurement Type"="Measurement Type", "Sweep Mode"="Sweep Mode", "Force Mode"="Force Mode", "Maximum Force"="Maximum Force", "Step Size"="Step Size", "Compliance"="Compliance", "Power Compliance"="Power Compliance", "Integration Time (s)"="Integration Time (s)") -> (w133:T70)
        n45 = call "TwoFourProbe.vi"("Sweeping Measurement"=w133, "Parameter Analizer in"=w132) -> ("Variant"=w153:variant, "Parameter Analizer out"=w131:T3)
        n46 = call "Edit Instruments Steps.vi"("Configuration"=w153, "error in (no error)"=w149, "Instrument"=Instrument_List."Parameter Analyzer", "Action"=Action."Configure", "Instrument Steps In"=w148) -> ("error out"=w150:errorcluster, "Instrument Steps Out"=w147:T58)  [unwired: 2 in, 2 out]
        n47 = Bundle By Name(cluster=w144, "Parameter Analyzer.Configuration"=w131) -> (w143:T1)
      }
      event "Configure Switching Matrix": Value Change {
        n48 = event-data() -> ()  [unwired: 2 out]
        n49 = Unbundle By Name(w157) -> ("Swithing Matrix.Configuration"=w166:T15)
        n50 = Bundle By Name(cluster=w166, "Connections"="Switching Matrix Connections") -> (w154:T15)
        n51 = To Variant(anything=w154) -> (Variant=w165:variant)
        n52 = Bundle By Name(cluster=w156, "Swithing Matrix.Configuration"=w154) -> (w155:T1)
        n53 = call "Edit Instruments Steps.vi"("Configuration"=w165, "error in (no error)"=w161, "Instrument"=Instrument_List."Switching Matrix", "Action"=Action."Configure", "Instrument Steps In"=w159) -> ("error out"=w162:errorcluster, "Instrument Steps Out"=w160:T58)  [unwired: 3 in, 1 out]
      }
      event "Configure Spectrometer": Value Change {
        n54 = event-data() -> ()  [unwired: 2 out]
        n55 = Unbundle By Name(w196) -> ("Switches & Mirrors.Configuration.Switches"=w176:T36, "Optical Spectrometer.Configuration"=w201:T23)
        n56 = case shown="\"Single Window\", Default" "Acquisition Mode" {
          tunnel: [enum16{"Single Window", "Multi-Window"}."Single Window" ("Optical Spectrometer.Acquisition Settings.Acquisition Mode") enum16{"Single Window", "Multi-Window"}."Multi-Window" ("Optical Spectrometer.Acquisition Settings.Acquisition Mode")] -> w181
          frame "Single Window", Default {
          }
          frame "Multi Window" {
          }
        }
        n57 = case shown="Default" "Power" {
          selector: "Power" -> [w214 _]
          tunnel: w201 -> [w216 w217]
          tunnel: [w215 w217] -> w178
          tunnel: w176 -> [w213 w221]
          tunnel: [w210 w218] -> w175
          frame Default {
            n58 = Bundle By Name(cluster=w216, "Laser Settings.Neutral Density Filter"=w214) -> (w215:T23)
            n59 = Bundle By Name(cluster=w213, "Laser"=TRUE, "Video"=FALSE) -> (w210:T36)
          }
          frame "OFF" {
            n60 = Bundle By Name(cluster=w221, "Laser"=FALSE, "Video"=FALSE) -> (w218:T36)
          }
        }
        n61 = Bundle By Name(cluster=w178, "Laser Settings.Laser Wavelength"="Wavelength", "Spectrometer Settings.Confocal Hole Size (µm)"="Confocal Hole Size (µm)", "Spectrometer Settings.Grating"="Grating", "Spectrometer Settings.Detector"="Detector", "Acquisition Settings.Spectal Position (nm)"="Spectal Position (nm)", "Acquisition Settings.From (nm)"="From (nm)", "Acquisition Settings.To (nm)"="To (nm)", "Acquisition Settings.Integration Time (s)"="Spectrum Integration Time (s)", "Acquisition Settings.Number of Accumulations"="Number of Accumulations", "Acquisition Settings.AutoScanning"="AutoScanning", "Acquisition Settings.Spike Removal"="Spike Removal", "Acquisition Settings.Acquisition Mode"=w181) -> (w179:T23)
        n62 = Bundle("Configuration"=w179, "Switches"=w175) -> (w180:cluster{"Configuration":T23, "Switches":T36})  [unwired: 1 in]
        n63 = To Variant(anything=w180) -> (Variant=w200:variant)
        n64 = Bundle By Name(cluster=w195, "Switches & Mirrors.Configuration.Switches"=w175, "Optical Spectrometer.Configuration"=w179) -> (w194:T1)
        n65 = call "Edit Instruments Steps.vi"("Configuration"=w200, "error in (no error)"=w172, "Instrument"=Instrument_List."Optical Spectrometer", "Action"=Action."Configure", "Instrument Steps In"=w168) -> ("error out"=w173:errorcluster, "Instrument Steps Out"=w169:T58)  [unwired: 3 in, 1 out]
        n66 = case shown="True" "Focus" {
          tunnel: w169 -> [w203 w207]
          tunnel: w173 -> [w202 w206]
          tunnel: [w203 w205] -> w170
          tunnel: [w202 w204] -> w171
          frame False {
          }
          frame True {
            n67 = call "Edit Instruments Steps.vi"("error in (no error)"=w206, "Instrument"=Instrument_List."Autofocus", "Action"=Action."Configure", "Instrument Steps In"=w207) -> ("error out"=w204:errorcluster, "Instrument Steps Out"=w205:T58)  [unwired: 4 in, 1 out]
          }
        }
      }
      event Panel Close? {
        n68 = event-data() -> ()  [unwired: 5 out]
        n69 = Two Button Dialog(message="Do you really want to close this dialog?", 1:"No" ("F button name (\"Cancel\")"), 2:"Yes" ("T button name (\"OK\")")) -> (T button?=w228:bool)
        n70 = event-data("Discard?"=TRUE) -> ()  [unwired: 1 in, 1 out]
      }
      event "Delete Instrument Step": Value Change {
        n71 = event-data() -> ()  [unwired: 2 out]
        n72 = Delete From Array(array=w235, length=1, index="Step Index") -> (array with subset deleted=w234:T58)  [unwired: 1 out]
      }
    }
    n73 = Unbundle By Name(w23) -> ("Laser Settings.Laser Wavelength"=w37:T25, "Laser Settings.Neutral Density Filter"=w36:T26, "Spectrometer Settings.Confocal Hole Size (µm)"=w35:dbl, "Spectrometer Settings.Grating"=w34:T28, "Spectrometer Settings.Detector"=w33:T29, "Acquisition Settings.Spectal Position (nm)"=w32:dbl, "Acquisition Settings.From (nm)"=w31:dbl, "Acquisition Settings.To (nm)"=w30:dbl, "Acquisition Settings.Integration Time (s)"=w29:dbl, "Acquisition Settings.Number of Accumulations"=w28:i32, "Acquisition Settings.AutoScanning"=w27:bool, "Acquisition Settings.Spike Removal"=w26:bool, "Acquisition Settings.Acquisition Mode"=w24:enum16{"Single Window", "Multi-Window"})
    n74 = Select(t=T69."Enabled" ("Disabled"), s=w44, f=T69."Disabled and Grayed Out" ("Disabled")) -> (s? t:f=w41:T69)
    n75 = property on="Focus" class="Bool (strict)"("Value"=FALSE ("Focus"), "DisabledEnum"=w41) -> ()  [unwired: 2 in, 2 out]
    n76 = property on="Wavelength" class="Enum (strict)"("Value"=w37) -> ()  [unwired: 2 in, 2 out]
    n77 = case shown="\"Single Window\", Default" w24 {
      tunnel: [enum32{"Single Window", "Multi Window"}."Single Window" ("Acquisition Mode") enum32{"Single Window", "Multi Window"}."Multi Window" ("Acquisition Mode")] -> w25
      frame "Single Window", Default {
      }
      frame "Multi-Window" {
      }
    }
    n78 = property on="Power" class="Enum (strict)"("Value"=w36) -> ()  [unwired: 2 in, 2 out]
    n79 = property on="Confocal Hole Size (µm)" class="DigNum (strict)"("Value"=w35) -> ()  [unwired: 2 in, 2 out]
    n80 = property on="Grating" class="Ring (strict)"("Value"=w34) -> ()  [unwired: 2 in, 2 out]
    n81 = property on="Detector" class="Enum (strict)"("Value"=w33) -> ()  [unwired: 2 in, 2 out]
    n82 = property on="Spectal Position (nm)" class="DigNum (strict)"("Value"=w32) -> ()  [unwired: 2 in, 2 out]
    n83 = property on="From (nm)" class="DigNum (strict)"("Value"=w31) -> ()  [unwired: 2 in, 2 out]
    n84 = property on="To (nm)" class="DigNum (strict)"("Value"=w30) -> ()  [unwired: 2 in, 2 out]
    n85 = property on="Spectrum Integration Time (s)" class="DigNum (strict)"("Value"=w29) -> ()  [unwired: 2 in, 2 out]
    n86 = property on="Number of Accumulations" class="DigNum (strict)"("Value"=w28) -> ()  [unwired: 2 in, 2 out]
    n87 = property on="AutoScanning" class="Bool (strict)"("Value"=w27) -> ()  [unwired: 2 in, 2 out]
    n88 = property on="Spike Removal" class="Bool (strict)"("Value"=w26) -> ()  [unwired: 2 in, 2 out]
    n89 = property on="Acquisition Mode" class="TabCtl (strict)"("Value"=w25) -> ()  [unwired: 2 in, 2 out]
  }
  "Instrument Steps Out" <- w11
  n90 = case shown="\"Initialize\", Default" "Function" {
    tunnel: w6 -> [w243 w244]
    tunnel: [w240 w244] -> w5
    tunnel: w3 -> [w241 _]
    tunnel: w2 -> [w239 _]
    frame "Initialize", Default {
      n91 = Unregister For Events(event registration refnum=w241, error in=w243) -> (error out=w242:errorcluster)
      n92 = Destroy User Event(user event=w239, error in=w242) -> (error out=w240:errorcluster)
    }
    frame "Action" {
    }
  }
  "error out" <- w5
